vi "Oxford-1820-Main.vi"() -> ()   [LabVIEW 2013, in "Mercury iXX.lvlib"]
uses:
  <instrlib>/Mercury iXX/Mercury iXX.lvlib
  <instrlib>/Mercury iXX/Public/Controls/Unit String.ctl
  <instrlib>/Mercury iXX/Public/Libraries/Temperature/Controls/Temperature Device (Read).ctl
  <instrlib>/Mercury iXX/Public/Controls/Manufacturing Data.ctl
  <instrlib>/Mercury iXX/Public/Libraries/Temperature/Controls/Temperature Sensor Type.ctl
  <instrlib>/Mercury iXX/Public/Libraries/Temperature/Controls/Excitation Cluster.ctl
  <instrlib>/Mercury iXX/Public/Libraries/Temperature/Controls/Excitation Type.ctl
  <instrlib>/Mercury iXX/Public/Libraries/Temperature/Controls/Calibration Cluster.ctl
  <instrlib>/Mercury iXX/Public/Libraries/Temperature/Controls/Calibration Interpolation.ctl
  <instrlib>/Mercury iXX/Public/Libraries/Temperature/Controls/Loop Cluster.ctl
  <instrlib>/Mercury iXX/Public/Libraries/Temperature/Controls/Temperature Signals Cluster.ctl
  <instrlib>/Mercury iXX/Public/Libraries/Heater/Controls/Heater Device (Read).ctl
  <instrlib>/Mercury iXX/Public/Libraries/Heater/Controls/Heater Signals Cluster.ctl
  <instrlib>/Mercury iXX/Public/Libraries/Level Meter/Controls/Level Meter (Read).ctl
  <instrlib>/Mercury iXX/Public/Libraries/Level Meter/Controls/Nitrogen Configuration.ctl
  <instrlib>/Mercury iXX/Public/Libraries/Level Meter/Controls/Frequency Configuration.ctl
  <instrlib>/Mercury iXX/Public/Libraries/Level Meter/Controls/Signals.ctl
  <instrlib>/Mercury iXX/Public/Libraries/Level Meter/Controls/Helium Configuration.ctl
  <instrlib>/Mercury iXX/Public/Libraries/Level Meter/Controls/Resistance Configuration.ctl
  <instrlib>/Mercury iXX/Public/Libraries/Level Meter/Controls/Pre-Pulse.ctl
  <instrlib>/Mercury iXX/Public/Libraries/Level Meter/Controls/Pulse.ctl
  <instrlib>/Mercury iXX/Public/Libraries/Auxiliary/Controls/AUX Device (Read).ctl
  <instrlib>/Mercury iXX/Public/Libraries/Auxiliary/Controls/AUX Signals (Read).ctl
  <instrlib>/Mercury iXX/Public/Libraries/Magnet/Controls/Device (Read).ctl
  <instrlib>/Mercury iXX/Public/Libraries/Magnet/Controls/Signals (Read).ctl
  <instrlib>/Mercury iXX/Public/Libraries/Magnet/Controls/Identifier.ctl
  <instrlib>/Mercury iXX/Public/Libraries/Pressure/Controls/Pressure Device (Read).ctl
  <instrlib>/Mercury iXX/Public/Libraries/Pressure/Controls/Pressure Sensor Type.ctl
  <instrlib>/Mercury iXX/Public/Libraries/Pressure/Controls/Calibration Cluster.ctl
  <instrlib>/Mercury iXX/Public/Libraries/Pressure/Controls/Calibration Interpolation.ctl
  <instrlib>/Mercury iXX/Public/Libraries/Pressure/Controls/Loop Cluster.ctl
  <instrlib>/Mercury iXX/Public/Libraries/Pressure/Controls/Pressure Signals Cluster.ctl
  <instrlib>/Mercury iXX/Public/Libraries/Magnet/Controls/PSU Actions.ctl
  <instrlib>/Mercury iXX/Public/Libraries/Magnet/Controls/Switch Heater.ctl
  <instrlib>/Mercury iXX/Private/Controls/Command Verbs.ctl
  <instrlib>/Mercury iXX/Public/Controls/ISOBus Address.ctl
  <instrlib>/Mercury iXX/Public/Controls/Comms Transport Layer.ctl
  <instrlib>/Mercury iXX/Private/Controls/Query Dynamic Reference.ctl
  <instrlib>/Mercury iXX/Public/Controls/Mercury Reference.ctl
  <instrlib>/Mercury iXX/Public/Libraries/Magnet/Open/Open Magnet Device.vi
  <instrlib>/Mercury iXX/Public/Libraries/Magnet/Configuration/Set/PSU Action Status (Set).vi
  <instrlib>/Mercury iXX/Public/Libraries/Magnet/Signals/Read/Current (Read).vi
  <instrlib>/Mercury iXX/Public/Libraries/Magnet/Signals/Read/Persistant Current (Read).vi
  <instrlib>/Mercury iXX/Public/Libraries/Magnet/Signals/Read/Switch Heater Status (Read).vi
  <instrlib>/Mercury iXX/Public/Libraries/Magnet/Signals/Set/Switch Heater No Check (Set).vi
  <instrlib>/Mercury iXX/Public/Libraries/System/Read/Time (Read).vi
  <instrlib>/Mercury iXX/Public/Libraries/Magnet/Signals/Set/Target Field Rate (Set).vi
  <instrlib>/Mercury iXX/Public/Libraries/Magnet/Signals/Set/Target Field (Set).vi
  <instrlib>/Mercury iXX/Public/Libraries/Level Meter/Open/Open Level Meter Device.vi
  <instrlib>/Mercury iXX/Public/Libraries/Temperature/Open/Open Temperature Device.vi
  <userlib>/_OpenG.lib/error/error.llb/Filter Error Codes (Array)__ogtk.vi
  <instrlib>/Mercury iXX/Public/Libraries/System/Open/Open System.vi
  <instrlib>/Mercury iXX/Public/Libraries/System/Read/Catalogue (Read).vi
  <instrlib>/Mercury iXX/Public/Libraries/System/Read/Display Automatic Dimming (Read).vi
  <instrlib>/Mercury iXX/Public/Libraries/System/Read/Display Automatic Dimming Time (Read).vi
  <instrlib>/Mercury iXX/Public/Libraries/System/Read/Display Brightness (Read).vi
  <instrlib>/Mercury iXX/Public/Libraries/System/Read/Date (Read).vi
  <instrlib>/Mercury iXX/Public/Libraries/System/Read/DateTime (Read).vi
  <instrlib>/Mercury iXX/Public/Libraries/System/Read/HVer (Read).vi
  <instrlib>/Mercury iXX/Public/Libraries/System/Read/FVer (Read).vi
  <instrlib>/Mercury iXX/Public/Libraries/System/Read/Serial Number (Read).vi
  <instrlib>/Mercury iXX/Public/Libraries/System/Read/Flash Space (Read).vi
  <instrlib>/Mercury iXX/Public/Libraries/System/Read/Mode (Read).vi
  <instrlib>/Mercury iXX/Public/Libraries/System/Set/DateTime (Set).vi
  <instrlib>/Mercury iXX/Public/Libraries/Temperature/Configuration/Read/Serial Number (Read).vi
  <instrlib>/Mercury iXX/Public/Libraries/Temperature/Configuration/Read/Nickname (Read).vi
  <instrlib>/Mercury iXX/Public/Libraries/Temperature/Configuration/Read/Excitation Magnitude (Read).vi
  <instrlib>/Mercury iXX/Public/Libraries/Temperature/Configuration/Read/Temperature Sensor (Read).vi
  <instrlib>/Mercury iXX/Public/Libraries/Temperature/Configuration/Read/Excitation Type (Read).vi
  <instrlib>/Mercury iXX/Public/Libraries/Temperature/Configuration/Read/Calibration Hot Limit (Read).vi
  <instrlib>/Mercury iXX/Public/Libraries/Temperature/Configuration/Read/Calibration Cold Limit (Read).vi
  <instrlib>/Mercury iXX/Public/Libraries/Temperature/Signals/Read/Voltage (Read).vi
  <instrlib>/Mercury iXX/Public/Libraries/Temperature/Signals/Read/Temperature (Read).vi
  <instrlib>/Mercury iXX/Public/Libraries/Temperature/Configuration/Read/Temperature Device (Read).vi
  <instrlib>/Mercury iXX/Public/Libraries/Control Loop/Configuration/Read/Control Loop (Read).vi
  <instrlib>/Mercury iXX/Public/Libraries/Heater/Open/Open Heater Device.vi
  <instrlib>/Mercury iXX/Public/Libraries/Heater/Configuration/Read/Heater Device (Read).vi
  <instrlib>/Mercury iXX/Public/Libraries/Heater/Configuration/Read/Nickname (Read).vi
  <instrlib>/Mercury iXX/Public/Libraries/Heater/Configuration/Read/Serial Number (Read).vi
  <instrlib>/Mercury iXX/Public/Libraries/Heater/Configuration/Read/Voltage Limit (Read).vi
  <instrlib>/Mercury iXX/Public/Libraries/Heater/Configuration/Read/Nominal Resistance (Read).vi
  <instrlib>/Mercury iXX/Public/Libraries/Heater/Configuration/Read/Maximum Power (Read).vi
  <instrlib>/Mercury iXX/Public/Libraries/Heater/Signals/Read/Voltage (Read).vi
  <instrlib>/Mercury iXX/Public/Libraries/Heater/Signals/Read/Power (Read).vi
  <instrlib>/Mercury iXX/Public/Libraries/Heater/Signals/Read/Current (Read).vi
  <instrlib>/Mercury iXX/Public/Libraries/Auxiliary/Open/Open Auxiliary Device.vi
  <instrlib>/Mercury iXX/Public/Libraries/Auxiliary/Configuration/Read/Aux Device (Read).vi
  <instrlib>/Mercury iXX/Public/Libraries/Auxiliary/Configuration/Read/Serial Number (Read).vi
  <instrlib>/Mercury iXX/Public/Libraries/Auxiliary/Configuration/Read/Minimum Gas Flow (Read).vi
  <instrlib>/Mercury iXX/Public/Libraries/Auxiliary/Configuration/Read/Gas Flow Scaling (Read).vi
  <instrlib>/Mercury iXX/Public/Libraries/Auxiliary/Configuration/Read/Temperature Error Sensitivity (Read).vi
  <instrlib>/Mercury iXX/Public/Libraries/Auxiliary/Configuration/Read/Temperature Error Voltage Sensitivity (Read).vi
  <instrlib>/Mercury iXX/Public/Libraries/Auxiliary/Configuration/Read/Valve Gearing (Read).vi
  <instrlib>/Mercury iXX/Public/Libraries/Auxiliary/Configuration/Read/Stepper Speed (Read).vi
  <instrlib>/Mercury iXX/Public/Libraries/Auxiliary/Signals/Read/Position (Read).vi
  <instrlib>/Mercury iXX/Public/Libraries/Auxiliary/Signals/Read/Percent Open (Read).vi
  <instrlib>/Mercury iXX/Public/Libraries/Pressure/Open/Open Pressure Device.vi
  <instrlib>/Mercury iXX/Public/Libraries/Pressure/Configuration/Read/Pressure Device (Read).vi
  <instrlib>/Mercury iXX/Public/Libraries/Pressure/Configuration/Read/Nickname (Read).vi
  <instrlib>/Mercury iXX/Public/Libraries/Pressure/Signals/Read/Current (Read).vi
  <instrlib>/Mercury iXX/Public/Libraries/Pressure/Signals/Read/Voltage (Read).vi
  <instrlib>/Mercury iXX/Public/Libraries/Level Meter/Configuration/Read/Level Meter Device (Read).vi
  <instrlib>/Mercury iXX/Public/Libraries/Level Meter/Configuration/Read/Serial Number (Read).vi
  <instrlib>/Mercury iXX/Public/Libraries/Level Meter/Configuration/Read/Helium Probe Resistance (Read).vi
  <instrlib>/Mercury iXX/Public/Libraries/Level Meter/Configuration/Read/Helium Pulse Mag (Read).vi
  <instrlib>/Mercury iXX/Public/Libraries/Level Meter/Configuration/Read/Helium Pulse Duration (Read).vi
  <instrlib>/Mercury iXX/Public/Libraries/Level Meter/Configuration/Read/Nitrogen Freq at 100 (Read).vi
  <instrlib>/Mercury iXX/Public/Libraries/Level Meter/Configuration/Read/Nitrogen Pulse Count Period (Read).vi
  <instrlib>/Mercury iXX/Public/Libraries/Level Meter/Signals/Read/Probe Resistance Helium (Read).vi
  <instrlib>/Mercury iXX/Public/Libraries/Level Meter/Signals/Read/Probe Level Helium (Read).vi
  <instrlib>/Mercury iXX/Public/Libraries/Level Meter/Signals/Read/Probe Count Nitrogen (Read).vi
  <instrlib>/Mercury iXX/Public/Libraries/Level Meter/Signals/Read/Probe Level Nitrogen (Read).vi
  <instrlib>/Mercury iXX/Public/Libraries/Magnet/Configuration/Read/Magnet Device (Read).vi
  <instrlib>/Mercury iXX/Public/Libraries/Magnet/Configuration/Read/Serial Number (Read).vi
  <instrlib>/Mercury iXX/Public/Libraries/Magnet/Configuration/Read/Bipolar Output (Read).vi
  <instrlib>/Mercury iXX/Public/Libraries/Magnet/Configuration/Read/Output Configuration (Read).vi
  <instrlib>/Mercury iXX/Public/Libraries/Magnet/Configuration/Read/Current Limit (Read).vi
  <instrlib>/Mercury iXX/Public/Libraries/Magnet/Configuration/Read/Current to Field Factor (Read).vi
  <instrlib>/Mercury iXX/Public/Libraries/Magnet/Configuration/Read/Switch Present (Read).vi
  <instrlib>/Mercury iXX/Public/Libraries/Magnet/Configuration/Read/Software Voltage Limit (Read).vi
  <instrlib>/Mercury iXX/Public/Libraries/Magnet/Signals/Read/Current Rate (Read).vi
  <instrlib>/Mercury iXX/Public/Libraries/Magnet/Configuration/Read/PSU Action Status (Read).vi
  <instrlib>/Mercury iXX/Public/Libraries/Magnet/Signals/Read/Voltage (Read).vi
  <instrlib>/Mercury iXX/Public/Libraries/Magnet/Signals/Read/Field (Read).vi
  <instrlib>/Mercury iXX/Public/Libraries/Magnet/Signals/Read/Target Field Rate (Read).vi
  <instrlib>/Mercury iXX/Public/Libraries/Magnet/Signals/Read/Target Field (Read).vi
  <instrlib>/Mercury iXX/Public/Libraries/Magnet/Signals/Read/Persistant Field (Read).vi
  <instrlib>/Mercury iXX/Public/Libraries/Pressure.lvlib
  <instrlib>/Mercury iXX/Public/Libraries/System.lvlib
  <instrlib>/Mercury iXX/Public/Libraries/Control Loop.lvlib
  <instrlib>/Mercury iXX/Public/Libraries/Heater.lvlib
  <instrlib>/Mercury iXX/Public/Libraries/Temperature.lvlib
  <instrlib>/Mercury iXX/Public/Libraries/Auxiliary.lvlib
  <instrlib>/Mercury iXX/Public/Libraries/Magnet.lvlib
  <instrlib>/Mercury iXX/Public/Libraries/Level Meter.lvlib
  <instrlib>/Mercury iXX/Public/Libraries/System/Open/Open Device.vi
panel:
  out "LPF ON":timestamp
  in  "Tab Control":T1(tab)
  out "LPF Pressure":dbl format="%_5f mB"
  out "LPF Needle Valve (%)":dbl format="%_6g"
  out "LPF Temperature":dbl=4.2075 format="%_2f K"
  out "Magnet Temperature":dbl=3.8705 format="%_2f K"
  in  "Set Needle Valve (%)":dbl format="%_2g"
  out "He LVL Chart":dbl(slide)=52.0833 scale=0.0..100.0
  out "N2 LVL Chart":dbl(slide)=61.3025 scale=0.0..100.0
  out "Sentinel":bool=TRUE
  in  "Remote Mode":bool
  out "Power Supply Field (T)":dbl=0.0001 format="%#.5f"
  out "Magnet Field (T)":dbl format="%.5f"
  out "Voltage (V)":dbl=-0.0003 format="%.5f"
  out "Current (A)":dbl=0.0006 format="%.5f"
  out "N2 LEVEL":dbl=61.3025 format="%.0f %"
  out "He LEVEL":dbl=52.0833 format="%.0f %"
  in  "Fast/Slow Fill":bool
  in  "OK":bool
  out "Magnet Field (T)":dbl(knob) caption="Voltage (V)" scale=-20.0..20.0
  out "Magnet Status 2":string
  out "Switch Time":string="11:11:48"
  out "SWITCH HEATER":bool
  in  "PS Heat":bool
  in  "Clamp":bool
  in  "To Set":bool
  in  "To Zero":bool
  in  "Hold":bool
  out "Magnet Status":string="Clamped"
  out "Target Field Rate (T/min)":dbl=1.0 format="%.5f"
  out "Target Field (T)":dbl format="%#.5f"
  in  "Target Rate (T/min)":dbl=0.1 format="%.5f"
  in  "Target Field (T)":dbl format="%#.5f"
  in  "Send to IPS":bool
  out "Voltage (V)":dbl(knob)=-0.0003 scale=-10.0..10.0
  out "Current (A)":dbl(knob)=0.0006 scale=-180.0..180.0
  in  "Mercury Functions":T2(tab)=enum."Temperature"
  out "time stamp":timestamp=timestamp(3543841780 s since 1904-01-01)
  out "Free Space":i32=166384 caption="Free Space (KB)"
  out "Set Date Response":string="VALID"
  out "String":string="NORM" caption="User Mode"
  out "Date":string="2016:04:18"
  out "Time":string="11:29:40"
  out "Hardware Version":string="65"
  out "Firmware Version":string="2.2.6.20"
  out "Serial Number":string="154650110"
  out "ITC Devices":string[](array[string])=["DB4.G1:AUX", "DB8.P1:PRES", "MB0.H1:HTR", "MB1.T1:TEMP"]
  out "S/W Version(s)":string[](array[string])=["2.2.6.20\n"]
  out "Serial Number(s)":string[](array[string])=["154650110"]
  out "# of Instruments":i32=1
  out "Automatic Dimming":string="OFF"
  out "Dimming Time":string="5"
  out "Display Brightness":string="100"
  in  "ITC IP Address":string="130.49.180.101"
  out "Excitation Magnitude":dbl=5.0
  out "Sensor Type":string="NTC"
  out "Excitation Type":string="UNIP"
  out "Hot Limit":dbl=1000.0
  out "H Unit":T3="K"
  out "Cold Limit":dbl=1000.0
  out "C Unit":T3="K"
  out "Unit":T3
  out "Voltage":dbl=0.005
  out "V Unit":T3="V"
  out "Temperature":dbl=4.2075
  out "T Unit":T3="K"
  out "Temperature Device Settings":T4={"Manufacturing"={"Hardware Version"="65", "Firmware Version"="2.2", "Serial Number"="154650110"}, "Temperature Sensor Type"="NTC", "Excitation"={"Excitation Type"="UNIP", "Magnitude"="5.00"}, "Calibration"={"Filename"="59543_iTC-lambda.dat", "Interpolation"="LIN", "Scaling Factor"="1", "Offset Factor"="0", "Hot Limit"="1000.00K", "Cold Limit"="1000.00K", "Last Calibration"="", "Reference"="Internal"}, "Control Loop"={"Heater"="", "Auxiliary"="", "Heater Auto"="", "Percentage Heat"="", "Temperature Set Point"="", "PID Auto (from file)"="", "P Value"="", "I Value"="", "D Value"="", "Auto PID Table Filename"="", "Flow Auto"="", "Target Heater Table"="", "Sweep mode"="", "Sweep Table Filename"="", "Percentage Flow"=""}, "Temperature Signals"={"Voltage"="5.0000mV", "Current"="3.9694µA", "Power"="0.0199µW", "Resistance"="1259.6510R", "Temperature"="4.2075K", "Sensitivity"="299.3801R/K", "Reference"="N/A"}, "Nickname"="Mag_AB_MB1", "Status"="0"}
  out "Temp S/N":string="154650110"
  out "T Nickname":string="Mag_AB_MB1"
  out "T Loop Details":T11
  out "Heater Device Settings":T13={"Manufacturing"={"Hardware Version"="65", "Firmware Version"="2.3", "Serial Number"="154650110"}, "Nickname"="MB0.H1", "Voltage Limit"="1", "Nominal Resistance"="10", "Maximum Power"="0.1000", "Heater Signals"={"Voltage"="0.0507V", "Current"="-0.0000A", "Power"="0.0000W"}, "Status"="2"}
  out "Htr C Unit":T3="A"
  out "Htr P Unit":T3="W"
  out "Htr V Unit":T3="V"
  out "Htr Current":dbl=-0.0
  out "Htr Power":dbl
  out "Htr Voltage":dbl=0.0507
  out "Power Unit":T3
  out "Volt Unit":T3
  out "Res Unit":T3
  out "Maximum Power":dbl=0.1
  out "Htr Resistance":dbl=10.0
  out "Htr Voltage Limit":dbl=1.0
  out "Htr S/N":string="154650110"
  out "Htr Nickname":string="MB0.H1"
  out "Pressure Device":T15={"Manufacturing"={"Hardware Version"="3", "Firmware Version"="1.10", "Serial Number"="151150091"}, "Temperature Sensor Type"="RAT", "Calibration"={"Filename"="Lambda pressure control_10V ratiometric.dat", "Interpolation"="LIN", "Scaling Factor"="1", "Offset Factor"="-0.0004", "High Limit"="1000.00K", "Low Limit"="1000.00K", "Last Calibration"=""}, "Control Loop"={"Heater"="None", "Auxiliary"="None", "Heater Auto"="", "Percentage Heat"="", "Pressure Set Point"="", "PID Auto (from file)"="", "P Value"="", "I Value"="", "D Value"="1.0", "Auto PID Table Filename"="", "Flow Auto"="", "Target Heater Table"="", "Sweep mode"="", "Sweep Table Filename"="", "Percentage Flow"=""}, "Pressure Signals"={"Voltage"="-0.0822mV", "Current"="-0.0000A", "Power"="0.0000W", "Pressure"="0.0000mB"}, "Nickname"="Lam_P_DB8", "Status"="0"}
  out "Nickname":string="Lam_P_DB8"
  out "Current":dbl=-0.0
  out "Voltage":dbl=-8.219999999999999e-05
  out "Auxiliary Device Details":T21={"Manufacturing"={"Hardware Version"="65", "Firmware Version"="3.1", "Serial Number"="154650084"}, "Min Flow"=0.0, "Scaling Factor"=50.0, "Temp Err"=9.0, "Temp V Err"=11.0, "Gear"=2, "Speed"=2, "Signals"={"Position"=0.0, "% Open"=0.0, "I0"="ON", "I1"="OFF", "I2"="OFF", "I3"="OFF", "O0"="OFF", "O1"="OFF", "O2"="OFF", "O3"="OFF"}, "Nickname"="DB4.G1", "Status"="0"} {"Signals"."% Open" min=0.0 max=100.0 step=0.1 format="%.4f"; "Signals"."Position" max=20.0 step=1.0 format="%.4f"; "Speed" max=7 step=1; "Gear" max=7 step=1; "Temp V Err" min=0.0 max=20.0 step=0.1; "Temp Err" min=0.0 max=20.0 step=0.1; "Scaling Factor" min=0.0 max=99.0 step=0.1; "Min Flow" min=0.0 max=20.0 step=0.1}
  out "Aux S/N":string="154650084"
  out "Min Flow":dbl caption="Minimum Gas Flow" format="%#.1f"
  out "Scaling Factor":dbl=50.0 caption="Gas Flow Scaling Factor" format="%#.1f"
  out "Temp Err":dbl=9.0 caption="Temperature Error Sensitivity" format="%#.1f"
  out "Temp V Err":dbl=11.0 caption="Temperature Voltage Error Sensitivity" format="%#.1f"
  out "Gear":u32=2 caption="Valve Gearing"
  out "Speed":u32=2 caption="Stepper Speed"
  out "Unit 2":T3
  out "Unit 3":T3
  out "Unit 4":T3
  out "Unit 5":T3
  out "Unit 6":T3
  out "Unit 7":T3
  out "Position":u32
  out "% Open":dbl caption="Percentage Open (%)"
  out "Unit":T3
  out "Unit":T3="%"
  out "time stamp 2":timestamp=timestamp(3543841781 s since 1904-01-01)
  out "Free Space 2":i32=166316 caption="Free Space (KB)"
  out "Set Date Response 2":string="VALID"
  out "String 2":string="NORM" caption="User Mode"
  out "Date 2":string="2016:04:18"
  out "Time 2":string="11:29:45"
  out "Hardware Version 2":string="65"
  out "Firmware Version 2":string="2.2.6.20"
  out "Serial Number 2":string="153350063"
  out "IPS Devices":string[](array[string])=["DB3.L1:LVL", "GRPX:PSU", "GRPY:PSU", "GRPZ:PSU", "MB1.T1:TEMP", "PSU.M1:PSU", "PSU.M2:PSU", "PSU.M3:PSU"]
  out "S/W Version(s) 2":string[](array[string])=["2.2.6.20\n"]
  out "Serial Number(s) 2":string[](array[string])=["153350063"]
  out "# of Instruments 2":i32=1
  out "Automatic Dimming 2":string="OFF"
  out "Dimming Time 2":string="5"
  out "Display Brightness 2":string="100"
  in  "IPS IP Address":string="130.49.180.102"
  out "LVL Device DetailSettings":T23={"Manufacturing"={"Hardware Version"="65", "Firmware Version"="2.2", "Serial Number"="152450013"}, "Nitrogen Configuration"={"Frequency Configuration"={"Freq 0%"=0.0, "Freq 100%"=0.0}, "Pulse Period"=0.0}, "Signals"={"Helium Signals"={"Resistance"=75.5626, "Level"=52.0833}, "Nitrogen Signals"={"Count"=8800.0, "Freq"=487361.0, "Level"=61.3445}}, "Nickname"="DB3.L1", "Status"="0", "Helium Configuration"={"Resistance Configuration"={"Res 0%"=0.0, "Res 100%"=0.0}, "Pre-Pulse"={"Magnitude"=0.0, "Duration"=0.0}, "Pulse"={"Magnitude"=0.0, "Duration"=0.0, "Delay"=0.0}}}
  out "LVL S/N":string="152450013"
  out "LVL P Magnitude":dbl=125.0 caption="Pulse Magnitude (mA)"
  out "LVL P Duration":dbl=5.0 caption="Pulse Duration (s)"
  out "N Freq 100%":dbl=7880.0 caption="Frequency at 100% (Hz)"
  out "N Pulse Period":dbl=1000.0 caption="Pulse Period (ms)"
  out "He Res Config":T28={"Res 0%"=149.0, "Res 100%"=8.0}
  out "He Resistance":dbl=75.5626 caption="Resistance (Ohms)"
  out "He Level":dbl=52.0833 caption="Helium Level (%)"
  out "N Counter":u32 caption="Counter"
  out "N Level":dbl=61.3445 caption="Nitrogen Level (%)"
  out "Excitation Magnitude 2":dbl=5.0
  out "Sensor Type 2":string="NTC"
  out "Excitation Type 2":string="UNIP"
  out "Hot Limit 2":dbl=1000.0
  out "H Unit 2":T3="K"
  out "Cold Limit 2":dbl=1000.0
  out "C Unit 2":T3="K"
  out "Unit 12":T3
  out "Voltage 2":dbl=0.005
  out "V Unit 2":T3="V"
  out "Temperature 2":dbl=3.8706
  out "T Unit 2":T3="K"
  out "Temperature Device Settings 2":T4={"Manufacturing"={"Hardware Version"="65", "Firmware Version"="2.2", "Serial Number"="153350063"}, "Temperature Sensor Type"="NTC", "Excitation"={"Excitation Type"="UNIP", "Magnitude"="5.00"}, "Calibration"={"Filename"="Bob.dat", "Interpolation"="LIN", "Scaling Factor"="1", "Offset Factor"="0", "Hot Limit"="1000.00K", "Cold Limit"="1000.00K", "Last Calibration"="", "Reference"="Internal"}, "Control Loop"={"Heater"="", "Auxiliary"="", "Heater Auto"="", "Percentage Heat"="", "Temperature Set Point"="", "PID Auto (from file)"="", "P Value"="", "I Value"="", "D Value"="", "Auto PID Table Filename"="", "Flow Auto"="", "Target Heater Table"="", "Sweep mode"="", "Sweep Table Filename"="", "Percentage Flow"=""}, "Temperature Signals"={"Voltage"="5.0000mV", "Current"="3.5897µA", "Power"="0.0179µW", "Resistance"="1392.8897R", "Temperature"="3.8706K", "Sensitivity"="359.8580R/K", "Reference"="N/A"}, "Nickname"="MB1.T1", "Status"="0"}
  out "Temp S/N 2":string="153350063"
  out "T Nickname 2":string="MB1.T1"
  out "T Loop Details 2":T11
  out "Magnet Device Details":T31={"Manufacturing"={"Hardware Version"="NOT_FOUND", "Firmware Version"="NOT_FOUND", "Serial Number"="NOT_FOUND"}, "Nickname"="GRPZ", "Bipolar Output"="ON", "String"="PARA", "Current Limit"=174.0, "AtoB"=8.688, "Inductance"=39.406, "Switch Present"="PSU.M1", "Swh Htr Current"=86.0, "SW VLIM"=9.0, "V Trans Time"=1000.0, "Magnet PSU Signals"={"Voltage"=-0.0002, "Current"=0.0002, "Current Rate"=100.0, "Field"=0.0001, "Field Rate"=11.5101, "Persistant Current"=0.0003, "Persistant Field"=0.0, "Target Current"=0.0, "Target Field"=0.0, "Target Current Rate"=8.688, "Target Field Rate"=1.0, "Switch Heater Status (SWHT)"="OFF", "Switch Heater Status (SWHN)"="OFF"}, "PSU Action"="CLMP", "Status"="40000000", "Level Limit"=0.0, "Temperature Limit"=999.0} {"Temperature Limit" format="%#.1f"; "Level Limit" format="%#.1f"; "V Trans Time" format="%#.1f"; "SW VLIM" format="%#.1f"; "Swh Htr Current" format="%#.1f"; "Inductance" format="%#.1f"; "AtoB" format="%#.1f"; "Current Limit" format="%#.1f"}
  out "Mag S/N":string="NOT_FOUND"
  out "Bipolar Output":string="ON"
  out "Out Config":string="PARA" caption="Output Configuration"
  out "Current Limit":dbl=174.0 caption="Current Limit (A)" format="%#.1f"
  out "AtoB":dbl=8.688 caption="Current Field Factor (A/T)" format="%#.1f"
  out "Switch Present":string="PSU.M1"
  out "SW VLIM":dbl=9.0 caption="Software Voltage Limit (V)" format="%#.1f"
  out "Unit 8":T3
  out "Unit 9":T3
  out "Unit 10":T3
  out "Current Rate":dbl=100.0
  out "PSU Act Stat":string="CLMP" caption="PSU Action Status"
  out "Unit 11":T3="A/min"
  in  "Device Identifier":T33="GRPZ"
  out "Error List":T34(array[cluster])
  in  "Lambda":bool
  out "LPF on (s)":i32=5373
  # "Voltage (V)"
  # "Magnet (T)"
  # "Current (A)"
  # "Slow Rates\nCurrent Range (A)     Field Range (T)    Rate (T/min)\n0       -- 100        0    -- 11.5       0.91\n100     -- 150        11.5 -- 17.2       0.23\n150     -- 155.467    17.2 -- 18         0.11\n155.567 -- 172.471    18   -- 20         0.11\n\nFast Rates\nCurrent Range (A)     Field Range (T)    Rate (T/min)\n0       -- 155.467    0    -- 18         1.0\n155.567 -- 172.471    18   -- 20         0.25"
  # "ITC: 101\nIPS: 102\nIPS VR: 67"
  # "ITC: 101\nIPS: 102\nIPS VR: 67"
  # "This Control Doesn't Work"
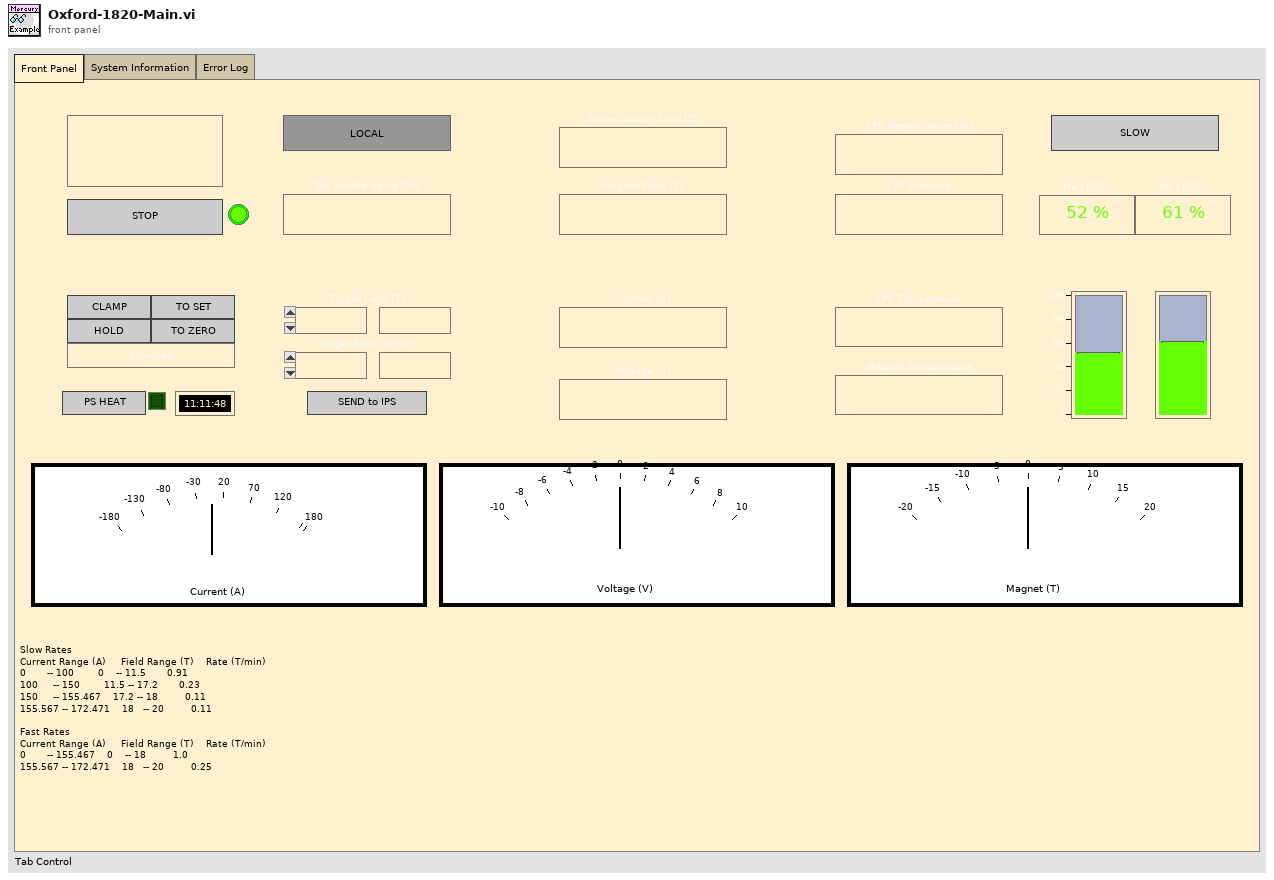
[diagram p1: front panel]
types:
  T1 = enum32{"Front Panel", "System Information", "Error Log"}
  T2 = enum32{"System: ITC", "Temperature", "Heater", "Pressure", "Auxiliary", "System: IPS", "Level Meter", "Temperature 2", "Magnet"}
  T3 = typedef "Mercury iXX.lvlib/Unit String.ctl" = string
  T4 = typedef "Mercury iXX.lvlib/Temperature.lvlib/Temperature Device (Read).ctl" = cluster{"Manufacturing":T5, "Temperature Sensor Type":T6, "Excitation":T7, "Calibration":T9, "Control Loop":T11, "Temperature Signals":T12, "Nickname":string, "Status":string}
  T5 = typedef "Mercury iXX.lvlib/Manufacturing Data.ctl" = cluster{"Hardware Version":string, "Firmware Version":string, "Serial Number":string}
  T6 = typedef "Mercury iXX.lvlib/Temperature.lvlib/Temperature Sensor Type.ctl" = string
  T7 = typedef "Mercury iXX.lvlib/Temperature.lvlib/Excitation Cluster.ctl" = cluster{"Excitation Type":T8, "Magnitude":string}
  T8 = typedef "Mercury iXX.lvlib/Temperature.lvlib/Excitation Type.ctl" = string
  T9 = typedef "Mercury iXX.lvlib/Temperature.lvlib/Calibration Cluster.ctl" = cluster{"Filename":string, "Interpolation":T10, "Scaling Factor":string, "Offset Factor":string, "Hot Limit":string, "Cold Limit":string, "Last Calibration":string, "Reference":string}
  T10 = typedef "Mercury iXX.lvlib/Temperature.lvlib/Calibration Interpolation.ctl" = string
  T11 = typedef "Mercury iXX.lvlib/Temperature.lvlib/Loop Cluster.ctl" = cluster{"Heater":string, "Auxiliary":string, "Heater Auto":string, "Percentage Heat":string, "Temperature Set Point":string, "PID Auto (from file)":string, "P Value":string, "I Value":string, "D Value":string, "Auto PID Table Filename":string, "Flow Auto":string, "Target Heater Table":string, "Sweep mode":string, "Sweep Table Filename":string, "Percentage Flow":string}
  T12 = typedef "Mercury iXX.lvlib/Temperature.lvlib/Temperature Signals Cluster.ctl" = cluster{"Voltage":string, "Current":string, "Power":string, "Resistance":string, "Temperature":string, "Sensitivity":string, "Reference":string}
  T13 = typedef "Mercury iXX.lvlib/Heater.lvlib/Heater Device (Read).ctl" = cluster{"Manufacturing":T5, "Nickname":string, "Voltage Limit":string, "Nominal Resistance":string, "Maximum Power":string, "Heater Signals":T14, "Status":string}
  T14 = typedef "Mercury iXX.lvlib/Heater.lvlib/Heater Signals Cluster.ctl" = cluster{"Voltage":string, "Current":string, "Power":string}
  T15 = typedef "Mercury iXX.lvlib/Pressure.lvlib/Pressure Device (Read).ctl" = cluster{"Manufacturing":T5, "Temperature Sensor Type":T16, "Calibration":T17, "Control Loop":T19, "Pressure Signals":T20, "Nickname":string, "Status":string}
  T16 = typedef "Mercury iXX.lvlib/Pressure.lvlib/Pressure Sensor Type.ctl" = string
  T17 = typedef "Mercury iXX.lvlib/Pressure.lvlib/Calibration Cluster.ctl" = cluster{"Filename":string, "Interpolation":T18, "Scaling Factor":string, "Offset Factor":string, "High Limit":string, "Low Limit":string, "Last Calibration":string}
  T18 = typedef "Mercury iXX.lvlib/Pressure.lvlib/Calibration Interpolation.ctl" = string
  T19 = typedef "Mercury iXX.lvlib/Pressure.lvlib/Loop Cluster.ctl" = cluster{"Heater":string, "Auxiliary":string, "Heater Auto":string, "Percentage Heat":string, "Pressure Set Point":string, "PID Auto (from file)":string, "P Value":string, "I Value":string, "D Value":string, "Auto PID Table Filename":string, "Flow Auto":string, "Target Heater Table":string, "Sweep mode":string, "Sweep Table Filename":string, "Percentage Flow":string}
  T20 = typedef "Mercury iXX.lvlib/Pressure.lvlib/Pressure Signals Cluster.ctl" = cluster{"Voltage":string, "Current":string, "Power":string, "Pressure":string}
  T21 = typedef "Mercury iXX.lvlib/Auxiliary.lvlib/AUX Device (Read).ctl" = cluster{"Manufacturing":T5, "Min Flow":dbl, "Scaling Factor":dbl, "Temp Err":dbl, "Temp V Err":dbl, "Gear":u32, "Speed":u32, "Signals":T22, "Nickname":string, "Status":string}
  T22 = typedef "Mercury iXX.lvlib/Auxiliary.lvlib/AUX Signals (Read).ctl" = cluster{"Position":dbl, "% Open":dbl, "I0":string, "I1":string, "I2":string, "I3":string, "O0":string, "O1":string, "O2":string, "O3":string}
  T23 = typedef "Mercury iXX.lvlib/Level Meter.lvlib/Level Meter (Read).ctl" = cluster{"Manufacturing":T5, "Nitrogen Configuration":T24, "Signals":T26, "Nickname":string, "Status":string, "Helium Configuration":T27}
  T24 = typedef "Mercury iXX.lvlib/Level Meter.lvlib/Nitrogen Configuration.ctl" = cluster{"Frequency Configuration":T25, "Pulse Period":dbl}
  T25 = typedef "Mercury iXX.lvlib/Level Meter.lvlib/Frequency Configuration.ctl" = cluster{"Freq 0%":dbl, "Freq 100%":dbl}
  T26 = typedef "Mercury iXX.lvlib/Level Meter.lvlib/Signals.ctl" = cluster{"Helium Signals":cluster{"Resistance":dbl, "Level":dbl}, "Nitrogen Signals":cluster{"Count":dbl, "Freq":dbl, "Level":dbl}}
  T27 = typedef "Mercury iXX.lvlib/Level Meter.lvlib/Helium Configuration.ctl" = cluster{"Resistance Configuration":T28, "Pre-Pulse":T29, "Pulse":T30}
  T28 = typedef "Mercury iXX.lvlib/Level Meter.lvlib/Resistance Configuration.ctl" = cluster{"Res 0%":dbl, "Res 100%":dbl}
  T29 = typedef "Mercury iXX.lvlib/Level Meter.lvlib/Pre-Pulse.ctl" = cluster{"Magnitude":dbl, "Duration":dbl}
  T30 = typedef "Mercury iXX.lvlib/Level Meter.lvlib/Pulse.ctl" = cluster{"Magnitude":dbl, "Duration":dbl, "Delay":dbl}
  T31 = typedef "Mercury iXX.lvlib/Magnet.lvlib/Device (Read).ctl" = cluster{"Manufacturing":T5, "Nickname":string, "Bipolar Output":string, "String":string, "Current Limit":dbl, "AtoB":dbl, "Inductance":dbl, "Switch Present":string, "Swh Htr Current":dbl, "SW VLIM":dbl, "V Trans Time":dbl, "Magnet PSU Signals":T32, "PSU Action":string, "Status":string, "Level Limit":dbl, "Temperature Limit":dbl}
  T32 = typedef "Mercury iXX.lvlib/Magnet.lvlib/Signals (Read).ctl" = cluster{"Voltage":dbl, "Current":dbl, "Current Rate":dbl, "Field":dbl, "Field Rate":dbl, "Persistant Current":dbl, "Persistant Field":dbl, "Target Current":dbl, "Target Field":dbl, "Target Current Rate":dbl, "Target Field Rate":dbl, "Switch Heater Status (SWHT)":string, "Switch Heater Status (SWHN)":string}
  T33 = typedef "Mercury iXX.lvlib/Magnet.lvlib/Identifier.ctl" = string
  T34 = cluster{"time":timestamp, "code":i32, "source":string}[]
  T35 = cluster{"Hold":bool, "Clamp":bool, "To Set":bool, "To Zero":bool, "Send to IPS":bool, "PS Heat":bool, "Lambda":bool}
  T36 = typedef "Mercury iXX.lvlib/Magnet.lvlib/PSU Actions.ctl" = string
  T37 = typedef "Mercury iXX.lvlib/Magnet.lvlib/Switch Heater.ctl" = string
  T38 = typedef "Mercury iXX.lvlib/Command Verbs.ctl" = string
  T39 = typedef "Mercury iXX.lvlib/ISOBus Address.ctl" = i32
  T40 = enum32{"invalid app kind", "Development System", "Run Time System", "Student Edition", "Embedded LabVIEW", "Evaluation", "Custom"}
  T41 = cluster{"time":timestamp, "code":i32, "source":string}
  T42 = enum32{"Invalid", "Standard", "Closed", "Hidden", "Minimized", "Maximized"}
  T43 = cluster{"Magnet Field":dbl, "PS Field":dbl, "Target Field":dbl, "Target Field Rate":dbl, "Voltage":dbl, "Current":dbl}
  T44 = typedef "Mercury iXX.lvlib/Comms Transport Layer.ctl" = enum16{"Ethernet TCP/IP", "USB", "ISOBus - RS-232", "GPIB"}
  T45 = typedef "Mercury iXX.lvlib/Query Dynamic Reference.ctl" = refnum<vi>
  T46 = typedef "Mercury iXX.lvlib/Mercury Reference.ctl" = cluster{"Comms":refnum<visa-resource-name>, "Device ID":string[], "Comms Layer":T44, "Command":string, "Query reference":T45}
  T47 = cluster{"Core":cluster{"Current VI Reference":refnum<vi>, "Close Panel on Exit?":bool}, "Mercury ITC Ref":cluster{"Comms":refnum<visa-resource-name>, "Device ID":string[], "Comms Layer":T44, "Command":string, "Query reference":T45}, "Mercury IPS Ref":T46, "sentinel":bool, "Error Log":cluster{"time":timestamp, "code":i32, "source":string}[]}
  T48 = typedef "Mercury iXX.lvlib/Response String.ctl" = string
  T49 = cluster{"Target Field (T)":dbl, "Target Field Rate (T/min)":dbl}
  T50 = cluster{"Comms":refnum<visa-resource-name>, "Device ID":string[], "Comms Layer":T44, "Command":string, "Query reference":T45}
  T51 = typedef "Filtered Error Details - Cluster__ogtk.ctl" = cluster{"code":i32, "source":string}
  T52 = cluster{"Current VI Reference":refnum<vi>, "Close Panel on Exit?":bool}
  T53 = typedef "Mercury iXX.lvlib/System.lvlib/User Mode.ctl" = string
  T54 = typedef "Mercury iXX.lvlib/Magnet.lvlib/Output Configuration.ctl" = string
  T55 = cluster{"Magnet Field":dbl, "PS Field":dbl, "Target Field":dbl, "Target Field Rate":dbl, "Voltage":dbl, "Current":dbl, "Switch":bool}
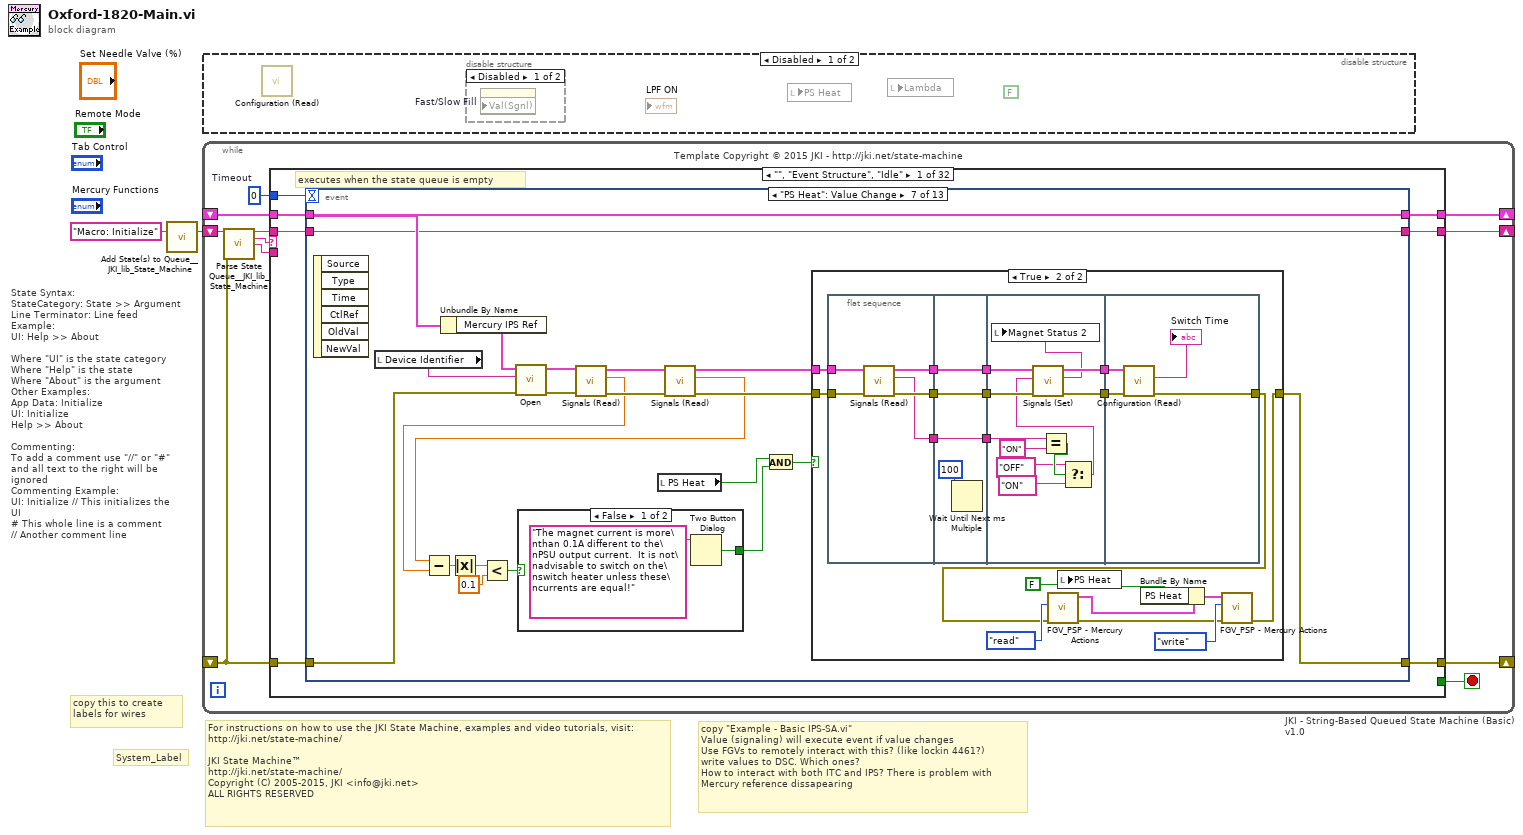
[diagram p0: block diagram]
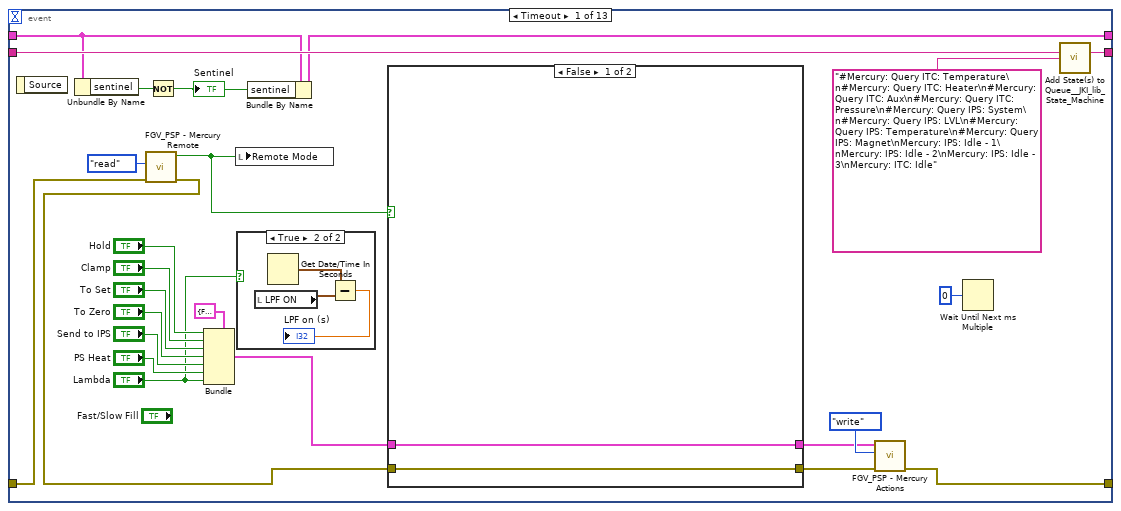
[diagram p4: hidden frame]
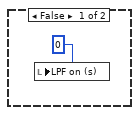
[diagram p5: hidden frame]
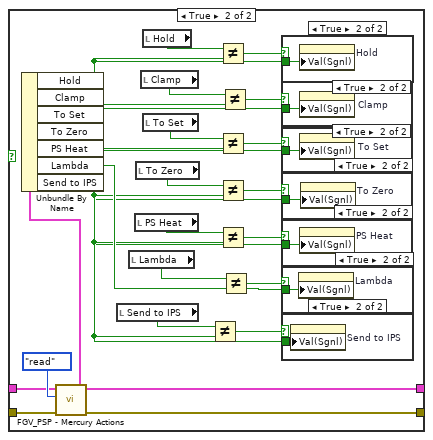
[diagram p6: hidden frame]
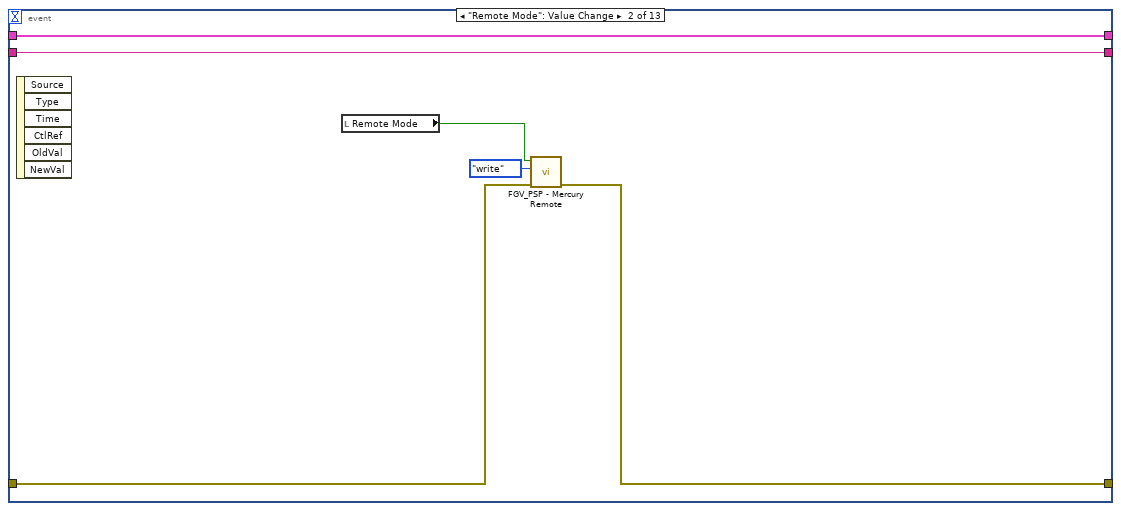
[diagram p14: hidden frame]
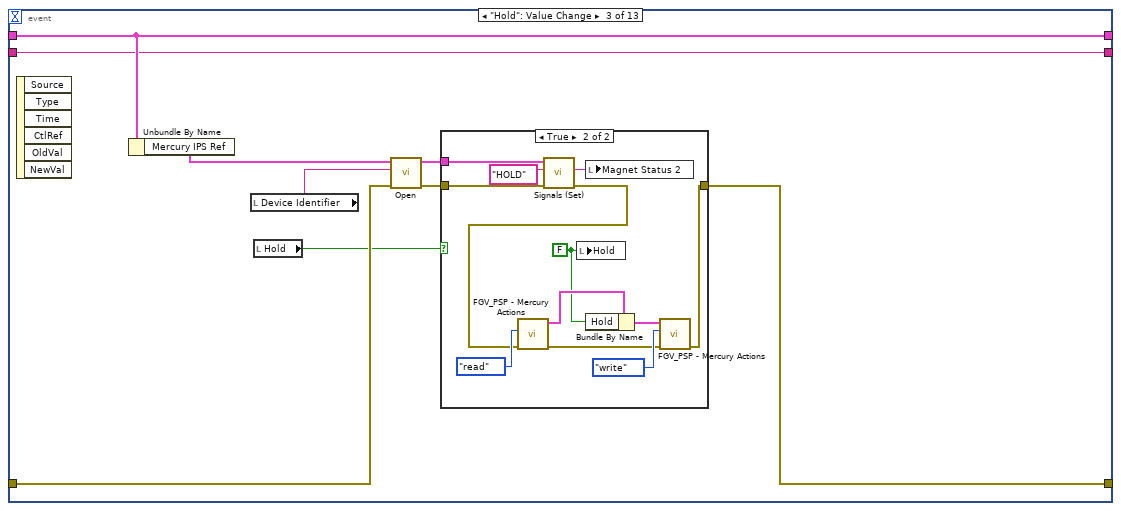
[diagram p15: hidden frame]
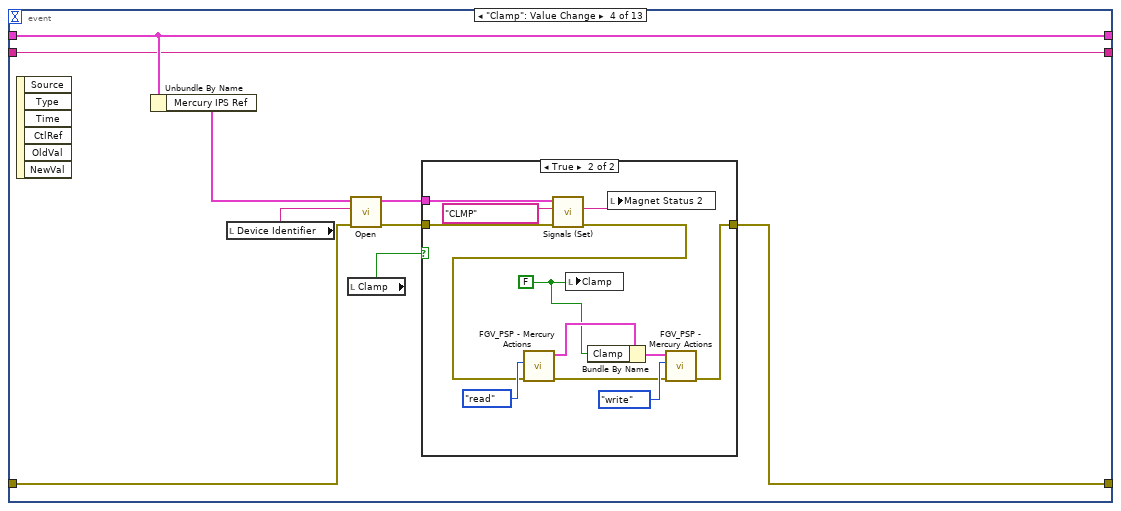
[diagram p17: hidden frame]
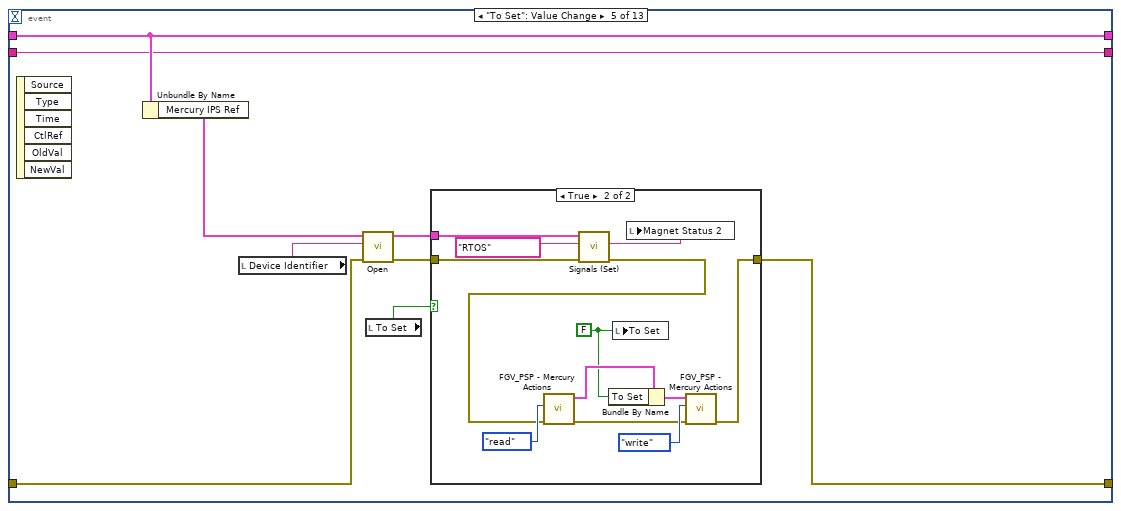
[diagram p19: hidden frame]
diagram:
  # "copy \"Example - Basic IPS-SA.vi\"\nValue (signaling) will execute event if value changes\nUse FGVs to remotely interact with this? (like lockin 4461?)\nwrite values to DSC. Which ones?\nHow to interact with both ITC and IPS? There is problem with \nMercury reference dissapearing"
  # "For instructions on how to use the JKI State Machine, examples and video tutorials, visit:\nhttp://jki.net/state-machine/\n\nJKI State Machine™\nhttp://jki.net/state-machine/\nCopyright (C) 2005-2015, JKI <info@jki.net>\nALL RIGHTS RESERVED"
  # "State Syntax:\nStateCategory: State >> Argument\nLine Terminator: Line feed\nExample:\nUI: Help >> About\n\nWhere \"UI\" is the state category\nWhere \"Help\" is the state\nWhere \"About\" is the argument\nOther Examples:\nApp Data: Initialize\nUI: Initialize\nHelp >> About\n\nCommenting:\nTo add a comment use \"//\" or \"#\" and all text to the right will be ignored\nCommenting Example:\nUI: Initialize // This initializes the UI\n# This whole line is a comment\n// Another comment line"
  # "copy this to create labels for wires"
  # "System_Label"
  n1 = call <vilib>:"Add State(s) to Queue__JKI_lib_State_Machine.vi"("State(s) in (\"\")"="Macro: Initialize") -> ("States Out"=w2:string)  [unwired: 14 in]
  n2 = while "JKI - String-Based Queued State Machine (Basic) v1.0" {
    shift-right: [w6] -> _
    shift-left: _ -> [w5]
    shift-right: [w9] -> _
    shift-left: _ -> [w3]
    shift-right: [w8] -> _
    shift-left: w2 -> [w10]
    stop <- w7 stop-if-true
    w4 = 0  # Timeout
    # "Template Copyright © 2015 JKI - http://jki.net/state-machine"
    n3 = call <vilib>:"Parse State Queue__JKI_lib_State_Machine.vi"("State Queue"=w10, "Error In (no error)"=w3) -> ("Remaining States"=w12:string, "Current State"=w13:string, "Arguments"=w11:string)  [unwired: 11 in]
    n4 = case shown="\"\", \"Event Structure\", \"Idle\"" w13 {
      selector: w13 -> [_ _ w361 _ _ _ _ _ _ _ _ _ _ _ _ _ _ _ _ _ _ _ _ _ _ _ _ _ _ _ _ _]
      tunnel: w12 -> [w20 w360 w365 w383 w400 w405 w409 w418 w424 w428 w440 w447 w458 w484 w489 w504 w508 w531 w575 w621 w663 w710 w731 w776 w817 w864 w905 w948 w1005 w1044 w1048 w1053]
      tunnel: w11 -> [_ _ _ _ _ _ _ _ _ _ _ w442 w452 _ _ _ _ _ _ _ _ _ _ _ _ _ _ _ _ _ _ _]
      tunnel: w5 -> [w16 w357 w363 w374 w386 w403 w406 _ w419 w425 w438 w445 w454 w481 w487 w502 w505 w526 w573 w620 w627 w670 w717 w774 w816 w863 w904 w947 w1004 w1043 w1047 w1052]
      tunnel: [w14 w358 w367 w380 errorcluster {"status"=FALSE, "code"=0, "source"=""} ("error out") w402 w407 w411 w420 w426 w434 w443 w455 w482 w486 w490 w506 w510 w535 w582 w624 w673 w718 w738 w783 w822 w871 w910 w982 w1017 w1046 w1050] -> w9
      tunnel: [w19 w359 w364 w382 w399 w404 w408 w417 w423 w427 w439 w446 w457 w483 w488 w503 w507 w530 w574 w622 w664 w711 w732 w775 w818 w865 w906 w949 w1006 w1045 w1049 w1054] -> w8
      tunnel: [_ _ _ _ _ TRUE _ _ _ _ _ _ _ _ _ _ _ _ _ _ _ _ _ _ _ _ _ _ _ _ _ _] -> w7
      tunnel: [w18 w357 w363 w381 w385 w403 w406 w416 w419 w425 w438 w445 w454 w481 w487 w502 w505 w525 w573 w620 w627 w670 w717 w774 w816 w863 w904 w947 w1004 w1043 w1047 w1052] -> w6
      tunnel: w4 -> [w17 _ _ _ _ _ _ _ _ _ _ _ _ _ _ _ _ _ _ _ _ _ _ _ _ _ _ _ _ _ _ _]
      tunnel: w3 -> [w15 w358 w366 w380 w395 w402 w407 w411 w421 w426 w430 w444 w456 w482 w486 w492 w506 w518 w537 w583 w630 w672 w712 w740 w785 w819 w866 w946 w983 w1018 w1046 w1051]
      frame "", "Event Structure", "Idle" {
        # "executes when the state queue is empty"
        n5 = event shown="[6] \"PS Heat\": Value Change" {
          selector: _ -> [_ _ _ _ _ _ _ _ _ _ _ _ _]
          dyn-events: _ -> [_ _ _ _ _ _ _ _ _ _ _ _ _]
          timeout: w17 -> [_ _ _ _ _ _ _ _ _ _ _ _ _]
          tunnel: w20 -> [w45 w87 w98 w120 w141 w164 w190 w254 w285 w326 w329 w350 w356]
          tunnel: [w44 w87 w98 w120 w141 w164 w190 w254 w285 w326 w329 w349 w355] -> w19
          tunnel: [w39 w86 w99 w121 w142 w163 w191 w250 w284 w318 w344 w347 w353] -> w18
          tunnel: w16 -> [w40 w86 w99 w121 w142 w163 w191 w250 w284 w318 w344 w347 w353]
          tunnel: w15 -> [w23 w89 w95 w116 w136 w158 w184 w253 w282 w323 w331 w348 w354]
          tunnel: [w33 w88 w97 w113 w143 w165 w189 w251 w281 w306 w332 w348 w354] -> w14
          event Timeout {
            n6 = event-data() -> ()  [unwired: 1 in, 1 out]
            n7 = Unbundle By Name(w40) -> ("sentinel"=w42:bool)
            n8 = call "FGV_PSP - Mercury Remote.vi"("error in"=w23, "Function"=enum16{"write", "read"}."read") -> ("error out"=w22:errorcluster, "Mercury Remote"=w21:bool)  [unwired: 4 in]
            n9 = Not(x=w42) -> (.not. x?=w41:bool)
            "Sentinel" <- w41
            n10 = Bundle(cluster=T35 {"Hold"=FALSE, "Clamp"=FALSE, "To Set"=FALSE, "To Zero"=FALSE, "Send to IPS"=FALSE, "PS Heat"=FALSE, "Lambda"=FALSE}, "Hold"="Hold", "Clamp"="Clamp", "To Set"="To Set", "To Zero"="To Zero", "Send to IPS"="Send to IPS", "PS Heat"="PS Heat", "Lambda"="Lambda") -> (w31:T35)
            n11 = local write "Remote Mode"(w21) -> ()
            n12 = case shown="True" "Lambda" {
              frame False {
                n13 = local write "LPF on (s)"(0 ("LPF on (s)")) -> ()
              }
              frame True {
                n14 = local read "LPF ON"() -> (w49:timestamp)
                n15 = Get Date/Time In Seconds() -> (seconds since 1Jan1904=w48:timestamp)
                n16 = Subtract(x=w48, y=w49) -> (x-y=→"LPF on (s)":dbl)
              }
            }
            n17 = Bundle By Name(cluster=w40, "sentinel"=w41) -> (w39:T47)
            n18 = case shown="False" w21 {
              tunnel: [w50 w76] -> w32
              tunnel: w22 -> [w50 w75]
              tunnel: w31 -> [w51 w74]
              tunnel: [w51 w66] -> w30
              frame False {
              }
              frame True {
                n19 = call "FGV_PSP - Mercury Actions.vi"("error in"=w75, "Function"=enum16{"write", "read"}."read", "mercury actions"=w74) -> ("error out"=w76:errorcluster, "mercury actions 2"=w66:T35)  [unwired: 3 in]
                n20 = Unbundle By Name(w66) -> ("Hold"=w58:bool, "Clamp"=w60:bool, "To Set"=w61:bool, "To Zero"=w62:bool, "PS Heat"=w63:bool, "Lambda"=w64:bool, "Send to IPS"=w65:bool)
                n21 = local read "Send to IPS"() -> (w59:bool)
                n22 = local read "Lambda"() -> (w57:bool)
                n23 = local read "PS Heat"() -> (w56:bool)
                n24 = local read "To Zero"() -> (w55:bool)
                n25 = local read "Clamp"() -> (w53:bool)
                n26 = local read "Hold"() -> (w52:bool)
                n27 = local read "To Set"() -> (w54:bool)
                n28 = Not Equal?(x=w59, y=w65) -> (x != y?=w67:bool)
                n29 = Not Equal?(x=w52, y=w58) -> (x != y?=w73:bool)
                n30 = Not Equal?(x=w54, y=w61) -> (x != y?=w71:bool)
                n31 = Not Equal?(x=w55, y=w62) -> (x != y?=w70:bool)
                n32 = Not Equal?(x=w56, y=w63) -> (x != y?=w69:bool)
                n33 = Not Equal?(x=w53, y=w60) -> (x != y?=w72:bool)
                n34 = Not Equal?(x=w57, y=w64) -> (x != y?=w68:bool)
                n35 = case shown="True" w73 {
                  tunnel: w58 -> [_ w84]
                  frame False {
                  }
                  frame True {
                    n36 = property on="Hold" class="Bool (strict)"("Val(Sgnl)"=w84) -> ()  [unwired: 2 in, 2 out]
                  }
                }
                n37 = case shown="True" w72 {
                  tunnel: w60 -> [_ w83]
                  frame False {
                  }
                  frame True {
                    n38 = property on="Clamp" class="Bool (strict)"("Val(Sgnl)"=w83) -> ()  [unwired: 2 in, 2 out]
                  }
                }
                n39 = case shown="True" w71 {
                  tunnel: w61 -> [_ w82]
                  frame False {
                  }
                  frame True {
                    n40 = property on="To Set" class="Bool (strict)"("Val(Sgnl)"=w82) -> ()  [unwired: 2 in, 2 out]
                  }
                }
                n41 = case shown="True" w70 {
                  tunnel: w62 -> [_ w81]
                  frame False {
                  }
                  frame True {
                    n42 = property on="To Zero" class="Bool (strict)"("Val(Sgnl)"=w81) -> ()  [unwired: 2 in, 2 out]
                  }
                }
                n43 = case shown="True" w69 {
                  tunnel: w63 -> [_ w80]
                  frame False {
                  }
                  frame True {
                    n44 = property on="PS Heat" class="Bool (strict)"("Val(Sgnl)"=w80) -> ()  [unwired: 2 in, 2 out]
                  }
                }
                n45 = case shown="True" w68 {
                  tunnel: w64 -> [_ w79]
                  frame False {
                  }
                  frame True {
                    n46 = property on="Lambda" class="Bool (strict)"("Val(Sgnl)"=w79) -> ()  [unwired: 2 in, 2 out]
                  }
                }
                n47 = case shown="True" w67 {
                  tunnel: w65 -> [_ w78]
                  frame False {
                  }
                  frame True {
                    n48 = property on="Send to IPS" class="Bool (strict)"("Val(Sgnl)"=w78) -> ()  [unwired: 2 in, 2 out]
                  }
                }
              }
            }
            n49 = call "FGV_PSP - Mercury Actions.vi"("error in"=w32, "Function"=enum16{"write", "read"}."write", "mercury actions"=w30) -> ("error out"=w33:errorcluster)  [unwired: 3 in, 1 out]
            n50 = Wait Until Next ms Multiple(millisecond multiple=u32 0) -> ()  [unwired: 1 out]
            n51 = call <vilib>:"Add State(s) to Queue__JKI_lib_State_Machine.vi"("State(s) in (\"\")"=w45, "State(s) at Back (\"\")"="#Mercury: Query ITC: Temperature\n#Mercury: Query ITC: Heater\n#Mercury: Query ITC: Aux\n#Mercury: Query ITC: Pressure\n#Mercury: Query IPS: System\n#Mercury: Query IPS: LVL\n#Mercury: Query IPS: Temperature\n#Mercury: Query IPS: Magnet\nMercury: IPS: Idle - 1\nMercury: IPS: Idle - 2\nMercury: IPS: Idle - 3\nMercury: ITC: Idle" ("State(s) at Back (\"\")")) -> ("States Out"=w44:string)  [unwired: 13 in]
          }
          event "Remote Mode": Value Change {
            n52 = event-data() -> ()  [unwired: 1 in, 6 out]
            n53 = local read "Remote Mode"() -> (w85:bool)
            n54 = call "FGV_PSP - Mercury Remote.vi"("error in"=w89, "Function"=enum16{"write", "read"}."write", "Mercury Remote"=w85) -> ("error out"=w88:errorcluster)  [unwired: 3 in, 1 out]
          }
          event "Hold": Value Change {
            n55 = event-data() -> ()  [unwired: 1 in, 6 out]
            n56 = Unbundle By Name(w99) -> ("Mercury IPS Ref"=w93:T46)
            n57 = local read "Device Identifier"() -> (w94:T33)
            n58 = local read "Hold"() -> (w91:bool)
            n59 = call-poly <instrlib>:"Open.vi"("error in (no error)"=w95, "Device Identifier"=w94, "Mercury Reference In"=w93) -> ("error out"=w96:errorcluster, "Mercury Reference Out"=w92:T46)  [unwired: 7 out]
            n60 = case shown="True" w91 {
              tunnel: [w100 w102] -> w97
              tunnel: w96 -> [w100 w111]
              tunnel: w92 -> [_ w110]
              frame False {
              }
              frame True {
                w107 = FALSE ("Hold")
                n61 = call-poly <instrlib>:"Signals (Set).vi"("error in"=w111, "PSU Act Stat"=T36 "HOLD", "Mercury Reference In"=w110) -> ("error out"=w101:errorcluster, "Response"=w109:T48)  [unwired: 1 in, 6 out]
                n62 = call "FGV_PSP - Mercury Actions.vi"("error in"=w101, "Function"=enum16{"write", "read"}."read") -> ("error out"=w104:errorcluster, "mercury actions 2"=w108:T35)  [unwired: 4 in]
                n63 = local write "Hold"(w107) -> ()
                n64 = local write "Magnet Status 2"(w109) -> ()
                n65 = Bundle By Name(cluster=w108, "Hold"=w107) -> (w106:T35)
                n66 = call "FGV_PSP - Mercury Actions.vi"("error in"=w104, "Function"=enum16{"write", "read"}."write", "mercury actions"=w106) -> ("error out"=w102:errorcluster)  [unwired: 3 in, 1 out]
              }
            }
          }
          event "Clamp": Value Change {
            n67 = event-data() -> ()  [unwired: 1 in, 6 out]
            n68 = Unbundle By Name(w121) -> ("Mercury IPS Ref"=w115:T46)
            n69 = local read "Device Identifier"() -> (w119:T33)
            n70 = local read "Clamp"() -> (w114:bool)
            n71 = call-poly <instrlib>:"Open.vi"("error in (no error)"=w116, "Device Identifier"=w119, "Mercury Reference In"=w115) -> ("error out"=w118:errorcluster, "Mercury Reference Out"=w117:T46)  [unwired: 7 out]
            n72 = case shown="True" w114 {
              tunnel: w118 -> [w122 w132]
              tunnel: w117 -> [_ w131]
              tunnel: [w122 w124] -> w113
              frame False {
              }
              frame True {
                w123 = FALSE
                n73 = call-poly <instrlib>:"Signals (Set).vi"("error in"=w132, "PSU Act Stat"=T36 "CLMP", "Mercury Reference In"=w131) -> ("error out"=w125:errorcluster, "Response"=w133:T48)  [unwired: 1 in, 6 out]
                n74 = call "FGV_PSP - Mercury Actions.vi"("error in"=w125, "Function"=enum16{"write", "read"}."read") -> ("error out"=w127:errorcluster, "mercury actions 2"=w130:T35)  [unwired: 4 in]
                n75 = local write "Clamp"(w123) -> ()
                n76 = Bundle By Name(cluster=w130, "Clamp"=w123) -> (w129:T35)
                n77 = local write "Magnet Status 2"(w133) -> ()
                n78 = call "FGV_PSP - Mercury Actions.vi"("error in"=w127, "Function"=enum16{"write", "read"}."write", "mercury actions"=w129) -> ("error out"=w124:errorcluster)  [unwired: 3 in, 1 out]
              }
            }
          }
          event "To Set": Value Change {
            n79 = event-data() -> ()  [unwired: 1 in, 6 out]
            n80 = Unbundle By Name(w142) -> ("Mercury IPS Ref"=w138:T46)
            n81 = local read "Device Identifier"() -> (w137:T33)
            n82 = call-poly <instrlib>:"Open.vi"("error in (no error)"=w136, "Device Identifier"=w137, "Mercury Reference In"=w138) -> ("error out"=w139:errorcluster, "Mercury Reference Out"=w140:T46)  [unwired: 7 out]
            n83 = local read "To Set"() -> (w135:bool)
            n84 = case shown="True" w135 {
              tunnel: [w144 w146] -> w143
              tunnel: w140 -> [_ w154]
              tunnel: w139 -> [w144 w153]
              frame False {
              }
              frame True {
                w145 = FALSE
                n85 = call-poly <instrlib>:"Signals (Set).vi"("error in"=w153, "PSU Act Stat"=T36 "RTOS", "Mercury Reference In"=w154) -> ("error out"=w147:errorcluster, "Response"=w155:T48)  [unwired: 1 in, 6 out]
                n86 = call "FGV_PSP - Mercury Actions.vi"("error in"=w147, "Function"=enum16{"write", "read"}."read") -> ("error out"=w149:errorcluster, "mercury actions 2"=w152:T35)  [unwired: 4 in]
                n87 = Bundle By Name(cluster=w152, "To Set"=w145) -> (w151:T35)
                n88 = local write "To Set"(w145) -> ()
                n89 = local write "Magnet Status 2"(w155) -> ()
                n90 = call "FGV_PSP - Mercury Actions.vi"("error in"=w149, "Function"=enum16{"write", "read"}."write", "mercury actions"=w151) -> ("error out"=w146:errorcluster)  [unwired: 3 in, 1 out]
              }
            }
          }
          event "To Zero": Value Change {
            n91 = event-data() -> ()  [unwired: 1 in, 6 out]
            n92 = Unbundle By Name(w163) -> ("Mercury IPS Ref"=w160:T46)
            n93 = local read "Device Identifier"() -> (w159:T33)
            n94 = local read "To Zero"() -> (w157:bool)
            n95 = call-poly <instrlib>:"Open.vi"("error in (no error)"=w158, "Device Identifier"=w159, "Mercury Reference In"=w160) -> ("error out"=w161:errorcluster, "Mercury Reference Out"=w162:T46)  [unwired: 7 out]
            n96 = case shown="True" w157 {
              tunnel: [w166 w169] -> w165
              tunnel: w162 -> [_ w176]
              tunnel: w161 -> [w166 w175]
              frame False {
              }
              frame True {
                w167 = FALSE
                n97 = call-poly <instrlib>:"Signals (Set).vi"("error in"=w175, "PSU Act Stat"=T36 "RTOZ", "Mercury Reference In"=w176) -> ("error out"=w170:errorcluster, "Response"=w177:T48)  [unwired: 1 in, 6 out]
                n98 = call "FGV_PSP - Mercury Actions.vi"("error in"=w170, "Function"=enum16{"write", "read"}."read") -> ("error out"=w172:errorcluster, "mercury actions 2"=w168:T35)  [unwired: 4 in]
                n99 = Bundle By Name(cluster=w168, "To Zero"=w167) -> (w174:T35)
                n100 = local write "To Zero"(w167) -> ()
                n101 = local write "Magnet Status 2"(w177) -> ()
                n102 = call "FGV_PSP - Mercury Actions.vi"("error in"=w172, "Function"=enum16{"write", "read"}."write", "mercury actions"=w174) -> ("error out"=w169:errorcluster)  [unwired: 3 in, 1 out]
              }
            }
          }
          event "PS Heat": Value Change {
            n103 = event-data() -> ()  [unwired: 1 in, 6 out]
            n104 = local read "Device Identifier"() -> (w185:T33)
            n105 = Unbundle By Name(w191) -> ("Mercury IPS Ref"=w187:T46)
            n106 = call-poly <instrlib>:"Open.vi"("error in (no error)"=w184, "Device Identifier"=w185, "Mercury Reference In"=w187) -> ("error out"=w181:errorcluster, "Mercury Reference Out"=w182:T46)  [unwired: 7 out]
            n107 = call-poly <instrlib>:"Signals (Read).vi"("error in"=w181, "Mercury Reference In"=w182) -> ("error out"=w193:errorcluster, "Current"=w188:dbl, "Mercury Reference Out"=w192:T46)  [unwired: 1 in, 6 out]
            n108 = local read "PS Heat"() -> (w180:bool)
            n109 = call-poly <instrlib>:"Signals (Read).vi"("error in"=w193, "Mercury Reference In"=w192) -> ("error out"=w194:errorcluster, "Persistant Current"=w183:dbl, "Mercury Reference Out"=w195:T46)  [unwired: 1 in, 6 out]
            n110 = Subtract(x=w183, y=w188) -> (x-y=w196:dbl)
            n111 = Absolute Value(x=w196) -> (abs(x)=w197:dbl)
            n112 = Less?(x=w197, y=0.1) -> (x < y?=w199:bool)
            n113 = case shown="False" w199 {
              selector: w199 -> [_ w202]
              tunnel: [w201 w202] -> w179
              frame False {
                n114 = Two Button Dialog(message="The magnet current is more\nthan 0.1A different to the\nPSU output current.  It is not\nadvisable to switch on the\nswitch heater unless these\ncurrents are equal!") -> (T button?=w201:bool)  [unwired: 2 out]
              }
              frame True {
              }
            }
            n115 = And(x=w180, y=w179) -> (x .and. y?=w186:bool)
            n116 = case shown="True" w186 {
              tunnel: w195 -> [_ w213]
              tunnel: w194 -> [w203 w212]
              tunnel: [w203 w204] -> w189
              frame False {
              }
              frame True {
                w206 = FALSE
                n117 = flat-sequence {
                  tunnel: [w224] -> w221
                  tunnel: [w223] -> w220
                  tunnel: [w222] -> w219
                  tunnel: w213 -> [w226]
                  tunnel: w212 -> [w225]
                  tunnel: w221 -> [w229]
                  tunnel: w220 -> [w228]
                  tunnel: [w229] -> w218
                  tunnel: [w228] -> w217
                  tunnel: [w227] -> w216
                  tunnel: w219 -> [w227]
                  tunnel: w218 -> [w240]
                  tunnel: w217 -> [w241]
                  tunnel: w216 -> [w238]
                  tunnel: [w235] -> w215
                  tunnel: [w236] -> w214
                  tunnel: w215 -> [w245]
                  tunnel: w214 -> [w244]
                  tunnel: [w243] -> w205
                  frame #0 {
                    n118 = call-poly <instrlib>:"Signals (Read).vi"("error in"=w225, "Mercury Reference In"=w226) -> ("error out"=w224:errorcluster, "Switch Heater Status"=w222:string, "Mercury Reference Out"=w223:T46)  [unwired: 1 in, 6 out]
                  }
                  frame #1 {
                    n119 = Wait Until Next ms Multiple(millisecond multiple=u32 100) -> ()  [unwired: 1 out]
                  }
                  frame #2 {
                    n120 = Equal?(x=w238, y="ON") -> (x = y?=w237:bool)
                    n121 = Select(t=T37 "OFF" ("Set Switch Heater"), s=w237, f=T37 "ON" ("Set Switch Heater")) -> (s? t:f=w232:T37)
                    n122 = call-poly <instrlib>:"Signals (Set).vi"("error in"=w240, "Set Switch Heater"=w232, "Mercury Reference In"=w241) -> ("error out"=w236:errorcluster, "Response"=w231:T48, "Mercury Reference Out"=w235:T46)  [unwired: 1 in, 5 out]
                    n123 = local write "Magnet Status 2"(w231) -> ()
                  }
                  frame #3 {
                    n124 = call-poly <instrlib>:"Configuration (Read).vi"("error in"=w244, "Mercury Reference In"=w245) -> ("error out"=w243:errorcluster, "Time"=→"Switch Time":string)  [unwired: 1 in, 7 out]
                  }
                }
                n125 = call "FGV_PSP - Mercury Actions.vi"("error in"=w205, "Function"=enum16{"write", "read"}."read") -> ("error out"=w209:errorcluster, "mercury actions 2"=w207:T35)  [unwired: 4 in]
                n126 = local write "PS Heat"(w206) -> ()
                n127 = Bundle By Name(cluster=w207, "PS Heat"=w206) -> (w211:T35)
                n128 = call "FGV_PSP - Mercury Actions.vi"("error in"=w209, "Function"=enum16{"write", "read"}."write", "mercury actions"=w211) -> ("error out"=w204:errorcluster)  [unwired: 3 in, 1 out]
              }
            }
          }
          event "Send to IPS": Value Change {
            n129 = event-data() -> ()  [unwired: 1 in, 6 out]
            n130 = local read "Device Identifier"() -> (w249:T33)
            n131 = Unbundle By Name(w250) -> ("Mercury IPS Ref"=w248:T46)
            n132 = local read "Send to IPS"() -> (w246:bool)
            n133 = call-poly <instrlib>:"Open.vi"("error in (no error)"=w253, "Device Identifier"=w249, "Mercury Reference In"=w248) -> ("error out"=w252:errorcluster, "Mercury Reference Out"=w247:T46)  [unwired: 7 out]
            n134 = case shown="True" w246 {
              tunnel: w252 -> [w255 w274]
              tunnel: [w255 w258] -> w251
              tunnel: w247 -> [_ w272]
              frame False {
              }
              frame True {
                w257 = FALSE
                n135 = local read "Remote Mode"() -> (w270:bool)
                n136 = case shown="True" w270 {
                  tunnel: "Target Field (T)" -> [w276 _]
                  tunnel: "Target Rate (T/min)" -> [w275 _]
                  tunnel: [w276 w278] -> w264
                  tunnel: [w275 w277] -> w265
                  frame False {
                  }
                  frame True {
                    n137 = call "FGV_PSP - Mercury Targets.vi"("Function"=enum16{"write", "read"}."read") -> ("Mercury Targets"=w279:T49)  [unwired: 5 in, 1 out]
                    n138 = Unbundle(w279) -> ("Target Field (T)"=w278:dbl, "Target Field Rate (T/min)"=w277:dbl)
                  }
                }
                n139 = local write "Send to IPS"(w257) -> ()
                n140 = call-poly <instrlib>:"Signals (Set).vi"("error in"=w274, "Target Field Rate"=w265, "Mercury Reference In"=w272) -> ("error out"=w273:errorcluster, "Mercury Reference Out"=w271:T46)  [unwired: 2 in, 5 out]
                n141 = local write "Target Field (T)"(w264) -> ()
                n142 = local write "Target Rate (T/min)"(w265) -> ()
                n143 = Bundle("Target Field (T)"=w264, "Target Field Rate (T/min)"=w265) -> (w267:T49)  [unwired: 1 in]
                n144 = call-poly <instrlib>:"Signals (Set).vi"("error in"=w273, "Target Field"=w264, "Mercury Reference In"=w271) -> ("error out"=w256:errorcluster)  [unwired: 2 in, 6 out]
                n145 = call "FGV_PSP - Mercury Actions.vi"("error in"=w256, "Function"=enum16{"write", "read"}."read") -> ("error out"=w261:errorcluster, "mercury actions 2"=w259:T35)  [unwired: 4 in]
                n146 = Bundle By Name(cluster=w259, "Send to IPS"=w257) -> (w263:T35)
                n147 = call "FGV_PSP - Mercury Actions.vi"("error in"=w261, "Function"=enum16{"write", "read"}."write", "mercury actions"=w263) -> ("error out"=w258:errorcluster)  [unwired: 3 in, 1 out]
                n148 = call "FGV_PSP - Mercury Targets.vi"("Function"=enum16{"write", "read"}."write", "Mercury Targets"=w267) -> ()  [unwired: 4 in, 2 out]
              }
            }
          }
          event "Lambda": Value Change {
            n149 = event-data() -> ()  [unwired: 1 in, 6 out]
            n150 = Unbundle By Name(w284) -> ("Mercury ITC Ref"=w283:T50)
            n151 = disable-structure shown="Disabled" {
              disable-tunnel: w283 -> [w302 _]
              disable-tunnel: w282 -> [w299 _]
              disable-tunnel: [w287 _] -> w281
              frame Disabled {
                # "TEMP device"
                # "AUX\nPRES\nHTR\nTEMP"
                n152 = local read "ITC Devices"() -> (w303:string[])
                n153 = Index Array(array=w303, index=3 ("Lambda device")) -> (element=w301:string)
                n154 = call-poly <instrlib>:"Open.vi"("error in (no error)"=w299, "Device Identifier"=w301, "Mercury Reference In"=w302) -> ("error out"=w291:errorcluster, "Mercury Reference Out"=w290:T46)  [unwired: 1 in, 6 out]
                n155 = local read "Lambda"() -> (w298:bool)
                n156 = call <instrlib>:"Build SCPI Command.vi"("error in"=w291, "Noun(s)"=":SIG:PERC:", "Verb"=T38 "SET:", "Mercury Reference In"=w290) -> ("error out"=w288:errorcluster, "SCPI Message(s)"=w292:string[], "Mercury Reference Out"=w294:T46)  [unwired: 5 in]
                n157 = Select(t="ON" ("Sweep Mode"), s=w298, f="OFF" ("Sweep Mode")) -> ()  [unwired: 1 out]
                n158 = case shown="True" w298 {
                  frame False {
                    n159 = local write "LPF ON"(timestamp(0 s since 1904-01-01) ("LPF ON")) -> ()
                  }
                  frame True {
                    n160 = Get Date/Time In Seconds() -> (seconds since 1Jan1904=w305:timestamp)
                    n161 = local write "LPF ON"(w305) -> ()
                  }
                }
                n162 = call <instrlib>:"Set (Str).vi"("ISOBUS address"=T39 -1, "error in"=w288, "SCPI Message(s)"=w292, "Mercury Reference In"=w294) -> ("error out"=w287:errorcluster, "Response"=w286:T48)  [unwired: 4 in, 2 out]
                n163 = local write "Magnet Status 2"(w286) -> ()
              }
              frame Enabled {
              }
            }
          }
          event "Fast/Slow Fill": Value Change {
            n164 = event-data() -> ()  [unwired: 1 in, 6 out]
            n165 = local read "IPS Devices"() -> (w320:string[])
            n166 = Unbundle By Name(w318) -> ("Mercury IPS Ref"=w325:T46)
            n167 = Index Array(array=w320, index=0) -> (element=w319:string)
            n168 = call-poly <instrlib>:"Open.vi"("error in (no error)"=w323, "Device Identifier"=w319, "Mercury Reference In"=w325) -> ("error out"=w316:errorcluster, "Mercury Reference Out"=w324:T46)  [unwired: 7 out]
            n169 = local read "Fast/Slow Fill"() -> (w311:bool)
            n170 = call <instrlib>:"Build SCPI Command.vi"("error in"=w316, "Noun(s)"=":HEL:PULS:SLOW:", "Verb"=T38 "SET:", "Mercury Reference In"=w324) -> ("error out"=w309:errorcluster, "SCPI Message(s)"=w314:string[], "Mercury Reference Out"=w308:T46)  [unwired: 5 in]
            n171 = Select(t="OFF" ("Temperature setpoint"), s=w311, f="ON" ("Temperature setpoint")) -> (s? t:f=w313:string)
            n172 = call <instrlib>:"Set (Str).vi"("ISOBUS address"=T39 -1, "error in"=w309, "Command Value (Str)"=w313, "SCPI Message(s)"=w314, "Mercury Reference In"=w308) -> ("error out"=w306:errorcluster, "Response"=w307:T48)  [unwired: 5 out]
            n173 = local write "Magnet Status 2"(w307) -> ()
          }
          event "Set Needle Valve (%)": Value Change {
            n174 = event-data() -> ("NewVal"=w333:dbl)  [unwired: 1 in, 5 out]
            n175 = Unbundle By Name(w344) -> ("Mercury ITC Ref"=w345:T50)
            n176 = local read "ITC Devices"() -> (w342:string[])
            n177 = Index Array(array=w342, index=3) -> (element=w341:string)
            n178 = call-poly <instrlib>:"Open.vi"("error in (no error)"=w331, "Device Identifier"=w341, "Mercury Reference In"=w345) -> ("error out"=w335:errorcluster, "Mercury Reference Out"=w334:T46)  [unwired: 7 out]
            n179 = call <instrlib>:"Build SCPI Command.vi"("error in"=w335, "Noun(s)"=":LOOP:FSET:", "Verb"=T38 "SET:", "Mercury Reference In"=w334) -> ("error out"=w336:errorcluster, "SCPI Message(s)"=w327:string[], "Mercury Reference Out"=w338:T46)  [unwired: 5 in]
            n180 = call <instrlib>:"Set (DBL).vi"("ISOBUS address"=T39 -1, "Unit"=T3 "", "error in"=w336, "Command Value (Dbl)"=w333, "SCPI Message(s)"=w327, "Mercury Reference In"=w338) -> ("error out"=w332:errorcluster, "Response"=w328:T48)  [unwired: 2 in, 2 out]
            n181 = local write "Magnet Status 2"(w328) -> ()
          }
          event "OK": Value Change {
            # "Exit Button Value Change (pressed) Event\n(this executes Macro: Exit to terminate the VI)"
            n182 = event-data() -> ()  [unwired: 1 in, 1 out]
            n183 = call <vilib>:"Add State(s) to Queue__JKI_lib_State_Machine.vi"("State(s) in Front (\"\")"="Macro: Exit", "State(s) in (\"\")"=w350) -> ("States Out"=w349:string)  [unwired: 13 in]
          }
          event Panel Close? {
            # "Discard the event because we'll close the front panel ourselves in Macro: Exit"
            # "Close Panel button (pressed) Event\n(this executes Macro: Exit to terminate the VI)"
            n184 = event-data() -> ()  [unwired: 1 in, 1 out]
            n185 = call <vilib>:"Add State(s) to Queue__JKI_lib_State_Machine.vi"("State(s) in Front (\"\")"="Macro: Exit", "State(s) in (\"\")"=w356) -> ("States Out"=w355:string)  [unwired: 13 in]
            n186 = event-data("Discard?"=TRUE) -> ()  [unwired: 1 in, 1 out]
          }
        }
      }
      frame "---------- Core ----------" {
        # "Do not put any code in this frame.\n(it is a separator no-op)"
        n187 = call <vilib>:"Add State(s) to Queue__JKI_lib_State_Machine.vi"("State(s) in (\"\")"=w360) -> ("States Out"=w359:string)  [unwired: 14 in]
      }
      frame Default {
        w370 = 42 items=["No error", "Argument error", "Memory is full", "Out of zone", "End of file", "File already open", "Generic file I/O error", "File not found", "File permission error", "Disk is full", "Duplicate path", "Too many files open", "System feature not enabled", "Resource file not found", "Cannot add resource", "Resource not found", "Image not found", "Image memory error", "Pen does not exist", "Config type invalid", "Config token not found", "Config parse error", "Config memory error", "Bad external code format", "Bad external code offset", "External code not present", "Null window", "Destroy window error", "Null menu", "Print aborted", "Bad print record", "Print driver error", "Windows error during printing", "Memory error during printing", "Print dialog error", "Generic print error", "Invalid device refnum", "Device not found", "Device parameter error", "Device unit error", "Cannot open device", "Device call aborted", "Generic error", "Cancelled by user", "Object ID too low", "Object ID too high", "Object not in heap", "Unknown heap", "Unknown object (invalid DefProc)", "Unknown object (DefProc not in table)", "Message out of range", "Invalid (null) method", "Unknown message", "Manager call not supported", "Bad address", "Network operation in progress", "Network operation timed out", "Connection is busy", "Network attribute not supported", "Network error", "Address in use", "System out of memory", "Connection aborted", "Connection refused", "Not connected", "Already connected", "Connection closed", "Initialization error (interapplication manager)", "Bad occurrence", "Wait on unbound occurrence handler", "Occurrence queue overflow", "Datalog type conflict", "Unused", "Unrecognized type (interapplication manager)", "Memory corrupt", "Failed to make temporary DLL", "Old CIN version", "Drag socket not found", "Failed to load drop-object", "Failed to register OLE object", "Failed to release OLE object", "Format specifier type mismatch", "Unknown format specifier", "Too few format specifiers", "Too many format specifiers", "Scan failed", "Newer CIN version", "Error converting to variant", "Runtime menu error", "Password tampered", "Variant attribute not found", "Incompatible variant data type", "Event data is not available", "Event Store is not present", "Occurrence is not found", "Event Queue is not created", "Event info is not available", "Refnum passed is NULL", "Error retrieving Class GUID", "Error retrieving CoClass GUID", "Error retrieving TypeLib GUID.", "Bad built application magic bytes.", "Specific driver is different from the specific driver associated with the Logical Name.", "There is no session opened to the class driver.", "Max Error", "MAX - Error with config objects", "MAX - Error loading configuration", "MAX - Group not supported"]
        # "Current State"
        # "Do not delete, rename, or modify this frame.\n(this is used to capture unhandled states and typos)"
        # "Handle mistyped state name (developer tool)"
        n188 = Format Into String(format string="Software Exception: Unhandled State \"%s\"." ("message"), error in=w366, w361) -> (resulting string=w369:string, error out=w368:errorcluster)  [unwired: 1 in]
        n189 = call <vilib>:"Error Cluster From Error Code.vi"("show call chain? (False)"=TRUE, "error in (no error)"=w368, "error message (\"\")"=w369, "error code (0)"=w370) -> ("error out"=w367:errorcluster)  [unwired: 5 in]
        n190 = call <vilib>:"Add State(s) to Queue__JKI_lib_State_Machine.vi"("State(s) in (\"\")"=w365) -> ("States Out"=w364:string)  [unwired: 14 in]
      }
      frame "Initialize Core Data" {
        # "Do not delete, rename, or modify this frame.\n(this is used to determine panel behavior on exit)"
        # "originally closed?"
        # "exe?"
        # "If panel starts closed or is an EXE, then close it when we exit"
        n191 = property class="VI"() -> ("Front Panel.Open"=w379:bool)  [unwired: 2 in, 2 out]
        n192 = property class="App"() -> ("App.Kind"=w378:T40)  [unwired: 2 in, 2 out]
        n193 = control-ref of="Current VI Reference"() -> (w372:refnum<vi>)
        n194 = Not(x=w379) -> (.not. x?=w376:bool)
        n195 = Equal?(x=w378, y=T40."Run Time System" ("Application:Kind")) -> (x = y?=w375:bool)
        n196 = Or(x=w376, y=w375) -> (x .or. y?=w373:bool)
        n197 = Bundle By Name(cluster=w374, "Core.Current VI Reference"=w372, "Core.Close Panel on Exit?"=w373) -> (w381:T47)
        n198 = call <vilib>:"Add State(s) to Queue__JKI_lib_State_Machine.vi"("State(s) in (\"\")"=w383) -> ("States Out"=w382:string)  [unwired: 14 in]
      }
      frame "Error Handler" {
        w394 = i32[] [-1950679035, -1950678943]  # Error Codes to Filter
        # "Unhandled Error -- Display it"
        # "Handle any errors here.\nYou can also output any states to clean-up after errors occur"
        # "Clear error"
        n199 = call-poly <userlib>:"Filter Error Codes__ogtk.vi"("Error In"=w395, "Error Codes to Filter"=w394) -> ("Error Out"=w396:errorcluster, "Filtered Error Details"=w393:T51)  [unwired: 7 in, 1 out]
        n200 = Unbundle(w393) -> ("code"=w391:i32, "source"=w392:string)
        n201 = Get Date/Time In Seconds() -> (seconds since 1Jan1904=w390:timestamp)
        n202 = Unbundle By Name(w386) -> ("Error Log"=w388:T34)
        n203 = Bundle By Name(cluster=T41 {"time"=timestamp(0 s since 1904-01-01), "code"=0, "source"=""} ("output cluster"), "time"=w390, "code"=w391, "source"=w392) -> (w387:T41)
        n204 = Build Array (concatenate)(w388, w387) -> (w384:T34)
        "Error List" <- w384
        n205 = Bundle By Name(cluster=w386, "Error Log"=w384) -> (w385:T47)
        n206 = call <vilib>:"General Error Handler.vi"("error in (no error)"=w396) -> ()  [unwired: 10 in, 5 out]
        n207 = call <vilib>:"Add State(s) to Queue__JKI_lib_State_Machine.vi"("State(s) in Front (\"\")"="/* Post Error States", "State(s) in (\"\")"=w400) -> ("States Out"=w399:string)  [unwired: 13 in]
      }
      frame "Exit" {
        # "Do not put any code in this frame.\n(No errors that occur here will be handled.)"
        n208 = call <vilib>:"Add State(s) to Queue__JKI_lib_State_Machine.vi"("State(s) in (\"\")"=w405) -> ("States Out"=w404:string)  [unwired: 14 in]
      }
      frame "---------- Data ----------" {
        # "Do not put any code in this frame.\n(It is a separator no-op. You can make a copy of this frame to create a new Data frame)"
        n209 = call <vilib>:"Add State(s) to Queue__JKI_lib_State_Machine.vi"("State(s) in (\"\")"=w409) -> ("States Out"=w408:string)  [unwired: 14 in]
      }
      frame "Data: Initialize" {
        w410 = T34 []  # Error Log
        w412 = TRUE  # sentinel
        w413 = T46 {"Comms"="", "Device ID"=[], "Comms Layer"=enum."Ethernet TCP/IP", "Command"="", "Query reference"=refnum}  # Mercury IPS Ref
        w414 = T50 {"Comms"="", "Device ID"=[], "Comms Layer"=enum."Ethernet TCP/IP", "Command"="", "Query reference"=refnum}  # Mercury ITC Ref
        w415 = T52 {"Current VI Reference"=refnum, "Close Panel on Exit?"=FALSE}  # Core
        # "do not delete - used by framework"
        # "Expand Bundle to add new data elements to shift register data."
        # "Add new data here."
        # "Data names and types of shift register data are defined by this bundle."
        # "Initialize the shift-register data, here.\n(data names are defined by what you wire into the bundle function)"
        n210 = Bundle("Core"=w415, "Mercury ITC Ref"=w414, "Mercury IPS Ref"=w413, "sentinel"=w412, "Error Log"=w410) -> (w416:T47)  [unwired: 1 in]
        n211 = call <vilib>:"Add State(s) to Queue__JKI_lib_State_Machine.vi"("State(s) in (\"\")"=w418) -> ("States Out"=w417:string)  [unwired: 14 in]
      }
      frame "Data: Cleanup" {
        # "Cleanup any data and references, here.\n(this is called automatically, by the Macro: Exit)"
        n212 = Unbundle By Name(w419) -> ("Core.Current VI Reference"=w422:refnum<vi>)
        n213 = Close Reference(reference=w422, error in (no error)=w421) -> (error out=w420:errorcluster)
        n214 = call <vilib>:"Add State(s) to Queue__JKI_lib_State_Machine.vi"("State(s) in (\"\")"=w424) -> ("States Out"=w423:string)  [unwired: 14 in]
      }
      frame "---------- UI ----------" {
        # "Do not put any code in this frame.\n(It is a separator no-op. You can make a copy of this frame to create a new UI frame)"
        n215 = call <vilib>:"Add State(s) to Queue__JKI_lib_State_Machine.vi"("State(s) in (\"\")"=w428) -> ("States Out"=w427:string)  [unwired: 14 in]
      }
      frame "UI: Initialize" {
        w435 = FALSE
        # "start in local mode"
        # "Initialize the User Interface, here.\n(this is called automatically, by the Macro: Init)"
        n216 = disable-structure shown="Disabled" {
          frame Disabled {
            n217 = Open VI Reference(vi path=path "") -> ()  [unwired: 5 in, 2 out]
            n218 = call "MNK_Dashboard_v2.vi"() -> ()  [unwired: 12 in]
          }
          frame Enabled {
          }
        }
        n219 = Open Application Reference(8:w430) -> (0:w432:errorcluster, 3:w433:refnum<vi>)  [unwired: 3 in]
        n220 = property class="App"(reference=w433, error in=w432, "WebSrvr.Active"=TRUE ("Web Server:Server Active")) -> (error out=w429:errorcluster)  [unwired: 1 out]
        n221 = call <vilib>:"Add State(s) to Queue__JKI_lib_State_Machine.vi"("State(s) in (\"\")"=w440) -> ("States Out"=w439:string)  [unwired: 14 in]
        n222 = local write "Remote Mode"(w435) -> ()
        n223 = call "FGV - Attocube Remote.vi"("error in"=w429, "Function"=enum16{"write", "read"}."write", "Attocube Remote"=w435) -> ("error out"=w434:errorcluster)  [unwired: 3 in, 1 out]
        "Magnet Status 2" <- "" ("Magnet Status 2")
      }
      frame "UI: Cursor Set" {
        # "Argument"
        # "Set and Unset Cursor Busy.\n(Usage: \"UI: Cursor Set >> Busy|Idle\")"
        n224 = case shown="\"Idle\", Default" w442 {
          tunnel: w444 -> [w449 w451]
          tunnel: [w448 w450] -> w443
          frame "Idle", Default {
            n225 = call <vilib>:"Unset Busy.vi"("error in (no error)"=w449) -> ("error out"=w448:errorcluster)  [unwired: 10 in]
          }
          frame "Busy" {
            n226 = call <vilib>:"Set Busy.vi"("error in (no error)"=w451) -> ("error out"=w450:errorcluster)  [unwired: 9 in, 1 out]
          }
        }
        n227 = call <vilib>:"Add State(s) to Queue__JKI_lib_State_Machine.vi"("State(s) in (\"\")"=w447) -> ("States Out"=w446:string)  [unwired: 14 in]
      }
      frame "UI: Front Panel State" {
        # "Argument"
        # "Set Front Panel Open or Closed\n(Usage: \"UI: Front Panel State >> Open|Close\")"
        n228 = Unbundle By Name(w454) -> ("Core.Current VI Reference"=w453:refnum<vi>)
        n229 = case shown="\"Open\", Default" w452 {
          tunnel: w456 -> [w462 w475]
          tunnel: [w464 w476] -> w455
          tunnel: w453 -> [w463 w473]
          frame "Open", Default {
            n230 = property class="VI"(reference=w463, error in=w462) -> (reference out=w460:refnum<vi>, error out=w461:errorcluster, "Front Panel.Open"=w459:bool)
            n231 = case shown="True" w459 {
              tunnel: [w467 w470] -> w464
              tunnel: w461 -> [w466 w470]
              tunnel: w460 -> [w465 _]
              frame False {
                n232 = invoke class="VI" method="FP.Open"(reference=w465, error in=w466, "Activate"=TRUE, "State"=T42."Standard") -> (error out=w467:errorcluster)  [unwired: 1 in, 4 out]
              }
              frame True {
              }
            }
          }
          frame "Close" {
            n233 = property class="VI"(reference=w473, error in=w475) -> (reference out=w472:refnum<vi>, error out=w474:errorcluster, "Front Panel.Open"=w471:bool)
            n234 = case shown="True" w471 {
              tunnel: [w477 w480] -> w476
              tunnel: w474 -> [w477 w479]
              tunnel: w472 -> [_ w478]
              frame False {
              }
              frame True {
                n235 = invoke class="VI" method="FP.Close"(reference=w478, error in=w479) -> (error out=w480:errorcluster)  [unwired: 1 in, 2 out]
              }
            }
          }
        }
        n236 = call <vilib>:"Add State(s) to Queue__JKI_lib_State_Machine.vi"("State(s) in (\"\")"=w458) -> ("States Out"=w457:string)  [unwired: 14 in]
      }
      frame "---------- Macro ----------" {
        # "Do not put any code in this frame.\n(It is a separator no-op. You can make a copy of this frame to create a new Macro frame)"
        n237 = call <vilib>:"Add State(s) to Queue__JKI_lib_State_Machine.vi"("State(s) in (\"\")"=w484) -> ("States Out"=w483:string)  [unwired: 14 in]
      }
      frame "Macro: Initialize" {
        w485 = "Data: Initialize\nInitialize Core Data\nUI: Initialize\nUI: Front Panel State >> Open\nMercury: Initialize"  # Data: Initialize Initialize Core Data UI: Initialize UI: Front Panel State >> Open Mercury: Initialize
        # "Initialization Macro\n(This is called once, when the VI starts)"
        n238 = call <vilib>:"Add State(s) to Queue__JKI_lib_State_Machine.vi"("State(s) in Front (\"\")"=w485, "State(s) in (\"\")"=w489) -> ("States Out"=w488:string)  [unwired: 13 in]
      }
      frame "Macro: Exit" {
        # "Exit Macro\n(This is called once, when the VI exits)"
        n239 = Unbundle By Name(w502) -> ("Core.Close Panel on Exit?"=w501:bool, "Mercury ITC Ref"=w494:T50, "Mercury IPS Ref"=w493:T46)
        n240 = call <instrlib>:"Close.vi"("error in (no error)"=w492, "Mercury Reference"=w493) -> ("error out"=w491:errorcluster)  [unwired: 9 out]
        n241 = call <instrlib>:"Close.vi"("error in (no error)"=w491, "Mercury Reference"=w494) -> ("error out"=w495:errorcluster)  [unwired: 9 out]
        n242 = call <vilib>:"Simple Error Handler.vi"("error in (no error)"=w495) -> ("error out"=w490:errorcluster)  [unwired: 1 in, 7 out]
        n243 = Select(t="UI: Front Panel State >> Close", s=w501, f="") -> (s? t:f=w498:string)
        n244 = call <vilib>:"Add State(s) to Queue__JKI_lib_State_Machine.vi"("State(s) in (\"\")"=w498, "State(s) at Back (\"\")"="Data: Cleanup\nExit") -> ("States Out"=w496:string)  [unwired: 13 in]
        n245 = call <vilib>:"Add State(s) to Queue__JKI_lib_State_Machine.vi"("State(s) in Front (\"\")"=w496, "State(s) in (\"\")"=w504) -> ("States Out"=w503:string)  [unwired: 13 in]
      }
      frame "---------- New Category ----------" {
        n246 = call <vilib>:"Add State(s) to Queue__JKI_lib_State_Machine.vi"("State(s) in (\"\")"=w508) -> ("States Out"=w507:string)  [unwired: 14 in]
      }
      frame "Mercury: Initialize" {
        w517 = Comms_Transport_Layer."Ethernet TCP/IP" ("Comms Layer")
        n247 = call-poly <instrlib>:"Open.vi"("Clear Previous Connections (False)"=TRUE ("Clear Previous Connections (True)"), "ID Query (True)"=TRUE, "IP Address"="ITC IP Address", "error in (no error)"=w518, "Comms Layer"=w517) -> ("error out"=w511:errorcluster, "# of Instruments"=→"# of Instruments":i32, "Serial Number(s)"=→"Serial Number(s)":string[], "Mercury Reference Out"=w512:T46, "S/W Version(s)"=→"S/W Version(s)":string[])  [unwired: 2 in]
        n248 = call-poly <instrlib>:"Open.vi"("Clear Previous Connections (False)"=FALSE ("Clear Previous Connections (True)"), "ID Query (True)"=TRUE, "IP Address"="IPS IP Address", "error in (no error)"=w511, "Comms Layer"=w517) -> ("error out"=w510:errorcluster, "# of Instruments"=→"# of Instruments 2":i32, "Serial Number(s)"=→"Serial Number(s) 2":string[], "Mercury Reference Out"=w509:T46, "S/W Version(s)"=→"S/W Version(s) 2":string[])  [unwired: 2 in]
        n249 = Bundle By Name(cluster=w526, "Mercury ITC Ref"=w512, "Mercury IPS Ref"=w509) -> (w525:T47)
        n250 = call <vilib>:"Add State(s) to Queue__JKI_lib_State_Machine.vi"("State(s) in (\"\")"=w531, "State(s) at Back (\"\")"="Mercury: Query ITC: System\nMercury: Query IPS: System\nMercury: Query ITC: Temperature\nMercury: Query ITC: Heater\nMercury: Query ITC: Aux\nMercury: Query ITC: Pressure\nMercury: Query IPS: LVL\nMercury: Query IPS: Temperature\nMercury: Query IPS: Magnet" ("State(s) at Back (\"\")")) -> ("States Out"=w530:string)  [unwired: 13 in]
      }
      frame "Mercury: Query ITC: System" {
        n251 = Unbundle By Name(w573) -> ("Mercury ITC Ref"=w533:T50)
        n252 = call-poly <instrlib>:"Configuration (Read).vi"("error in"=w537, "Mercury Reference In"=w533) -> ("error out"=w569:errorcluster, "Devices"=→"ITC Devices":string[], "Mercury Reference Out"=w570:T46)  [unwired: 1 in, 6 out]
        n253 = call-poly <instrlib>:"Configuration (Read).vi"("error in"=w569, "Mercury Reference In"=w570) -> ("error out"=w562:errorcluster, "Automatic Dimming"=→"Automatic Dimming":string, "Mercury Reference Out"=w563:T46)  [unwired: 1 in, 6 out]
        n254 = call-poly <instrlib>:"Configuration (Read).vi"("error in"=w562, "Mercury Reference In"=w563) -> ("error out"=w565:errorcluster, "Dimming Time"=→"Dimming Time":string, "Mercury Reference Out"=w564:T46)  [unwired: 1 in, 6 out]
        n255 = call-poly <instrlib>:"Configuration (Read).vi"("error in"=w565, "Mercury Reference In"=w564) -> ("error out"=w571:errorcluster, "Display Brightness"=→"Display Brightness":string, "Mercury Reference Out"=w572:T46)  [unwired: 1 in, 6 out]
        n256 = call-poly <instrlib>:"Configuration (Read).vi"("error in"=w571, "Mercury Reference In"=w572) -> ("error out"=w556:errorcluster, "Date"=→"Date":string, "Mercury Reference Out"=w555:T46)  [unwired: 1 in, 6 out]
        n257 = call-poly <instrlib>:"Configuration (Read).vi"("error in"=w556, "Mercury Reference In"=w555) -> ("error out"=w558:errorcluster, "Time"=→"Time":string, "Mercury Reference Out"=w557:T46)  [unwired: 1 in, 6 out]
        n258 = call-poly <instrlib>:"Configuration (Read).vi"("error in"=w558, "Mercury Reference In"=w557) -> ("error out"=w536:errorcluster, "time stamp"=→"time stamp":timestamp, "Mercury Reference Out"=w534:T46)  [unwired: 1 in, 6 out]
        n259 = call-poly <instrlib>:"Configuration (Read).vi"("error in"=w536, "Mercury Reference In"=w534) -> ("error out"=w554:errorcluster, "Hardware Version"=→"Hardware Version":string, "Mercury Reference Out"=w553:T46)  [unwired: 1 in, 6 out]
        n260 = call-poly <instrlib>:"Configuration (Read).vi"("error in"=w554, "Mercury Reference In"=w553) -> ("error out"=w552:errorcluster, "Firmware Version"=→"Firmware Version":string, "Mercury Reference Out"=w551:T46)  [unwired: 1 in, 6 out]
        n261 = call-poly <instrlib>:"Configuration (Read).vi"("error in"=w552, "Mercury Reference In"=w551) -> ("error out"=w539:errorcluster, "Serial Number"=→"Serial Number":string, "Mercury Reference Out"=w538:T46)  [unwired: 1 in, 6 out]
        n262 = call-poly <instrlib>:"Configuration (Read).vi"("error in"=w539, "Mercury Reference In"=w538) -> ("error out"=w545:errorcluster, "Free Space"=→"Free Space":i32, "Mercury Reference Out"=w544:T46)  [unwired: 1 in, 6 out]
        n263 = call-poly <instrlib>:"Configuration (Read).vi"("error in"=w545, "Mercury Reference In"=w544) -> ("error out"=w541:errorcluster, "Mode"=→"String":T53, "Mercury Reference Out"=w542:T46)  [unwired: 1 in, 6 out]
        n264 = Get Date/Time In Seconds() -> (seconds since 1Jan1904=w550:timestamp)
        n265 = call-poly <instrlib>:"Configuration (Set).vi"("error in"=w541, "time stamp"=w550, "Mercury Reference In"=w542) -> ("error out"=w535:errorcluster, "Response"=→"Set Date Response":T48)  [unwired: 1 in, 6 out]
        n266 = call <vilib>:"Add State(s) to Queue__JKI_lib_State_Machine.vi"("State(s) in (\"\")"=w575) -> ("States Out"=w574:string)  [unwired: 14 in]
      }
      frame "Mercury: Query ITC: Temperature" {
        # "Temperature"
        n267 = Unbundle By Name(w620) -> ("Mercury ITC Ref"=w577:T50)
        n268 = local read "ITC Devices"() -> (w576:string[])
        n269 = Index Array(array=w576, index=3) -> (element=w578:string)
        n270 = call-poly <instrlib>:"Open.vi"("error in (no error)"=w583, "Device Identifier"=w578, "Mercury Reference In"=w577) -> ("error out"=w595:errorcluster, "Mercury Reference Out"=w596:T46)  [unwired: 7 out]
        n271 = call-poly <instrlib>:"Configuration (Read).vi"("error in"=w595, "Mercury Reference In"=w596) -> ("error out"=w587:errorcluster, "Serial Number"=→"Temp S/N":string, "Mercury Reference Out"=w586:T46)  [unwired: 1 in, 6 out]
        n272 = call-poly <instrlib>:"Configuration (Read).vi"("error in"=w587, "Mercury Reference In"=w586) -> ("error out"=w589:errorcluster, "Nickname"=→"T Nickname":string, "Mercury Reference Out"=w588:T46)  [unwired: 1 in, 6 out]
        n273 = call-poly <instrlib>:"Configuration (Read).vi"("error in"=w589, "Mercury Reference In"=w588) -> ("error out"=w592:errorcluster, "Unit"=→"Unit":T3, "Excitation Magnitude"=→"Excitation Magnitude":dbl, "Mercury Reference Out"=w591:T46)  [unwired: 1 in, 5 out]
        n274 = call-poly <instrlib>:"Configuration (Read).vi"("error in"=w592, "Mercury Reference In"=w591) -> ("error out"=w581:errorcluster, "Sensor Type"=→"Sensor Type":T6, "Mercury Reference Out"=w579:T46)  [unwired: 1 in, 6 out]
        n275 = call-poly <instrlib>:"Configuration (Read).vi"("error in"=w581, "Mercury Reference In"=w579) -> ("error out"=w598:errorcluster, "Excitation Type"=→"Excitation Type":T8, "Mercury Reference Out"=w599:T46)  [unwired: 1 in, 6 out]
        n276 = call-poly <instrlib>:"Configuration (Read).vi"("error in"=w598, "Mercury Reference In"=w599) -> ("error out"=w600:errorcluster, "Unit"=→"H Unit":T3, "Hot Limit"=→"Hot Limit":dbl, "Mercury Reference Out"=w601:T46)  [unwired: 1 in, 5 out]
        n277 = call-poly <instrlib>:"Configuration (Read).vi"("error in"=w600, "Mercury Reference In"=w601) -> ("error out"=w607:errorcluster, "Unit"=→"C Unit":T3, "Cold Limit"=→"Cold Limit":dbl, "Mercury Reference Out"=w606:T46)  [unwired: 1 in, 5 out]
        n278 = call-poly <instrlib>:"Signals (Read).vi"("error in"=w607, "Mercury Reference In"=w606) -> ("error out"=w611:errorcluster, "Unit"=→"V Unit":T3, "Voltage"=→"Voltage":dbl, "Mercury Reference Out"=w610:T46)  [unwired: 1 in, 5 out]
        n279 = call-poly <instrlib>:"Signals (Read).vi"("error in"=w611, "Mercury Reference In"=w610) -> ("error out"=w612:errorcluster, "Unit"=→"T Unit":T3, "Temperature"=→"Temperature":dbl, "Mercury Reference Out"=w615:T46)  [unwired: 1 in, 5 out]
        n280 = call-poly <instrlib>:"Configuration (Read).vi"("error in"=w612, "Mercury Reference In"=w615) -> ("error out"=w618:errorcluster, "Device Details"=→"Temperature Device Settings":T4, "Mercury Reference Out"=w617:T46)  [unwired: 1 in, 6 out]
        n281 = call-poly <instrlib>:"Configuration (Read).vi"("error in"=w618, "Mercury Reference In"=w617) -> ("error out"=w582:errorcluster, "Loop Details"=→"T Loop Details":T11)  [unwired: 1 in, 7 out]
        n282 = call <vilib>:"Add State(s) to Queue__JKI_lib_State_Machine.vi"("State(s) in (\"\")"=w621) -> ("States Out"=w622:string)  [unwired: 14 in]
      }
      frame "Mercury: Query ITC: Heater" {
        # "Heater"
        n283 = Unbundle By Name(w627) -> ("Mercury ITC Ref"=w626:T50)
        n284 = local read "ITC Devices"() -> (w628:string[])
        n285 = Index Array(array=w628, index=2) -> (element=w623:string)
        n286 = call-poly <instrlib>:"Open.vi"("error in (no error)"=w630, "Device Identifier"=w623, "Mercury Reference In"=w626) -> ("error out"=w633:errorcluster, "Mercury Reference Out"=w632:T46)  [unwired: 7 out]
        n287 = call-poly <instrlib>:"Configuration (Read).vi"("error in"=w633, "Mercury Reference In"=w632) -> ("error out"=w640:errorcluster, "Device Details"=→"Heater Device Settings":T13, "Mercury Reference Out"=w639:T46)  [unwired: 1 in, 6 out]
        n288 = call-poly <instrlib>:"Configuration (Read).vi"("error in"=w640, "Mercury Reference In"=w639) -> ("error out"=w642:errorcluster, "Nickname"=→"Htr Nickname":string, "Mercury Reference Out"=w641:T46)  [unwired: 1 in, 6 out]
        n289 = call-poly <instrlib>:"Configuration (Read).vi"("error in"=w642, "Mercury Reference In"=w641) -> ("error out"=w635:errorcluster, "Serial Number"=→"Htr S/N":string, "Mercury Reference Out"=w634:T46)  [unwired: 1 in, 6 out]
        n290 = call-poly <instrlib>:"Configuration (Read).vi"("error in"=w635, "Mercury Reference In"=w634) -> ("error out"=w631:errorcluster, "Unit"=→"Volt Unit":T3, "Voltage Limit"=→"Htr Voltage Limit":dbl, "Mercury Reference Out"=w625:T46)  [unwired: 1 in, 5 out]
        n291 = call-poly <instrlib>:"Configuration (Read).vi"("error in"=w631, "Mercury Reference In"=w625) -> ("error out"=w645:errorcluster, "Unit"=→"Res Unit":T3, "Nominal Resistance"=→"Htr Resistance":dbl, "Mercury Reference Out"=w646:T46)  [unwired: 1 in, 5 out]
        n292 = call-poly <instrlib>:"Configuration (Read).vi"("error in"=w645, "Mercury Reference In"=w646) -> ("error out"=w652:errorcluster, "Unit"=→"Power Unit":T3, "Maximum Power"=→"Maximum Power":dbl, "Mercury Reference Out"=w651:T46)  [unwired: 1 in, 5 out]
        n293 = call-poly <instrlib>:"Signals (Read).vi"("error in"=w652, "Mercury Reference In"=w651) -> ("error out"=w654:errorcluster, "Unit"=→"Htr V Unit":T3, "Voltage"=→"Htr Voltage":dbl, "Mercury Reference Out"=w653:T46)  [unwired: 1 in, 5 out]
        n294 = call-poly <instrlib>:"Signals (Read).vi"("error in"=w654, "Mercury Reference In"=w653) -> ("error out"=w656:errorcluster, "Unit"=→"Htr P Unit":T3, "Power"=→"Htr Power":dbl, "Mercury Reference Out"=w655:T46)  [unwired: 1 in, 5 out]
        n295 = call-poly <instrlib>:"Signals (Read).vi"("error in"=w656, "Mercury Reference In"=w655) -> ("error out"=w624:errorcluster, "Unit"=→"Htr C Unit":T3, "Current"=→"Htr Current":dbl)  [unwired: 1 in, 6 out]
        n296 = call <vilib>:"Add State(s) to Queue__JKI_lib_State_Machine.vi"("State(s) in (\"\")"=w663) -> ("States Out"=w664:string)  [unwired: 14 in]
      }
      frame "Mercury: Query ITC: Aux" {
        # "Auxiliary"
        n297 = Unbundle By Name(w670) -> ("Mercury ITC Ref"=w665:T50)
        n298 = local read "ITC Devices"() -> (w668:string[])
        n299 = Index Array(array=w668, index=0) -> (element=w666:string)
        n300 = call-poly <instrlib>:"Open.vi"("error in (no error)"=w672, "Device Identifier"=w666, "Mercury Reference In"=w665) -> ("error out"=w692:errorcluster, "Mercury Reference Out"=w693:T46)  [unwired: 7 out]
        n301 = call-poly <instrlib>:"Configuration (Read).vi"("error in"=w692, "Mercury Reference In"=w693) -> ("error out"=w696:errorcluster, "Auxiliary Device Details"=→"Auxiliary Device Details":T21, "Mercury Reference Out"=w695:T46)  [unwired: 1 in, 6 out]
        n302 = call-poly <instrlib>:"Configuration (Read).vi"("error in"=w696, "Mercury Reference In"=w695) -> ("error out"=w699:errorcluster, "Serial Number"=→"Aux S/N":string, "Mercury Reference Out"=w698:T46)  [unwired: 1 in, 6 out]
        n303 = call-poly <instrlib>:"Configuration (Read).vi"("error in"=w699, "Mercury Reference In"=w698) -> ("error out"=w701:errorcluster, "Unit"=→"Unit 2":T3, "Min Flow"=→"Min Flow":dbl, "Mercury Reference Out"=w700:T46)  [unwired: 1 in, 5 out]
        n304 = call-poly <instrlib>:"Configuration (Read).vi"("error in"=w701, "Mercury Reference In"=w700) -> ("error out"=w703:errorcluster, "Unit"=→"Unit 3":T3, "Scaling Factor"=→"Scaling Factor":dbl, "Mercury Reference Out"=w702:T46)  [unwired: 1 in, 5 out]
        n305 = call-poly <instrlib>:"Configuration (Read).vi"("error in"=w703, "Mercury Reference In"=w702) -> ("error out"=w671:errorcluster, "Unit"=→"Unit 4":T3, "Temp Err"=→"Temp Err":dbl, "Mercury Reference Out"=w667:T46)  [unwired: 1 in, 5 out]
        n306 = call-poly <instrlib>:"Configuration (Read).vi"("error in"=w671, "Mercury Reference In"=w667) -> ("error out"=w675:errorcluster, "Unit"=→"Unit 5":T3, "Temp V Err"=→"Temp V Err":dbl, "Mercury Reference Out"=w674:T46)  [unwired: 1 in, 5 out]
        n307 = call-poly <instrlib>:"Configuration (Read).vi"("error in"=w675, "Mercury Reference In"=w674) -> ("error out"=w677:errorcluster, "Unit"=→"Unit 6":T3, "Gear"=→"Gear":u32, "Mercury Reference Out"=w676:T46)  [unwired: 1 in, 5 out]
        n308 = call-poly <instrlib>:"Configuration (Read).vi"("error in"=w677, "Mercury Reference In"=w676) -> ("error out"=w685:errorcluster, "Unit"=→"Unit 7":T3, "Speed"=→"Speed":u32, "Mercury Reference Out"=w684:T46)  [unwired: 1 in, 5 out]
        n309 = call-poly <instrlib>:"Signals (Read).vi"("error in"=w685, "Mercury Reference In"=w684) -> ("error out"=w687:errorcluster, "Unit"=→"Unit":T3, "Position"=→"Position":u32, "Mercury Reference Out"=w686:T46)  [unwired: 1 in, 5 out]
        n310 = call-poly <instrlib>:"Signals (Read).vi"("error in"=w687, "Mercury Reference In"=w686) -> ("error out"=w673:errorcluster, "Unit"=→"Unit":T3, "% Open"=→"% Open":dbl)  [unwired: 1 in, 6 out]
        n311 = call <vilib>:"Add State(s) to Queue__JKI_lib_State_Machine.vi"("State(s) in (\"\")"=w710) -> ("States Out"=w711:string)  [unwired: 14 in]
      }
      frame "Mercury: Query ITC: Pressure" {
        # "Pressure"
        n312 = Unbundle By Name(w717) -> ("Mercury ITC Ref"=w714:T50)
        n313 = local read "ITC Devices"() -> (w716:string[])
        n314 = Index Array(array=w716, index=1) -> (element=w713:string)
        n315 = call-poly <instrlib>:"Open.vi"("error in (no error)"=w712, "Device Identifier"=w713, "Mercury Reference In"=w714) -> ("error out"=w720:errorcluster, "Mercury Reference Out"=w721:T46)  [unwired: 7 out]
        n316 = call-poly <instrlib>:"Configuration (Read).vi"("error in"=w720, "Mercury Reference In"=w721) -> ("error out"=w722:errorcluster, "Device Details"=→"Pressure Device":T15, "Mercury Reference Out"=w723:T46)  [unwired: 1 in, 6 out]
        n317 = call-poly <instrlib>:"Configuration (Read).vi"("error in"=w722, "Mercury Reference In"=w723) -> ("error out"=w727:errorcluster, "Nickname"=→"Nickname":string, "Mercury Reference Out"=w728:T46)  [unwired: 1 in, 6 out]
        n318 = call-poly <instrlib>:"Signals (Read).vi"("error in"=w727, "Mercury Reference In"=w728) -> ("error out"=w725:errorcluster, "Current"=→"Current":dbl, "Mercury Reference Out"=w726:T46)  [unwired: 1 in, 6 out]
        n319 = call-poly <instrlib>:"Signals (Read).vi"("error in"=w725, "Mercury Reference In"=w726) -> ("error out"=w718:errorcluster, "Voltage"=→"Voltage":dbl)  [unwired: 1 in, 7 out]
        n320 = call <vilib>:"Add State(s) to Queue__JKI_lib_State_Machine.vi"("State(s) in (\"\")"=w731) -> ("States Out"=w732:string)  [unwired: 14 in]
      }
      frame "Mercury: Query IPS: System" {
        # "Your code here.\n(You can make a copy of, or modify, this frame)"
        n321 = Unbundle By Name(w774) -> ("Mercury IPS Ref"=w735:T46)
        n322 = call-poly <instrlib>:"Configuration (Read).vi"("error in"=w740, "Mercury Reference In"=w735) -> ("error out"=w760:errorcluster, "Devices"=→"IPS Devices":string[], "Mercury Reference Out"=w759:T46)  [unwired: 1 in, 6 out]
        n323 = call-poly <instrlib>:"Configuration (Read).vi"("error in"=w760, "Mercury Reference In"=w759) -> ("error out"=w764:errorcluster, "Automatic Dimming"=→"Automatic Dimming 2":string, "Mercury Reference Out"=w763:T46)  [unwired: 1 in, 6 out]
        n324 = call-poly <instrlib>:"Configuration (Read).vi"("error in"=w764, "Mercury Reference In"=w763) -> ("error out"=w761:errorcluster, "Dimming Time"=→"Dimming Time 2":string, "Mercury Reference Out"=w762:T46)  [unwired: 1 in, 6 out]
        n325 = call-poly <instrlib>:"Configuration (Read).vi"("error in"=w761, "Mercury Reference In"=w762) -> ("error out"=w758:errorcluster, "Display Brightness"=→"Display Brightness 2":string, "Mercury Reference Out"=w757:T46)  [unwired: 1 in, 6 out]
        n326 = call-poly <instrlib>:"Configuration (Read).vi"("error in"=w758, "Mercury Reference In"=w757) -> ("error out"=w767:errorcluster, "Date"=→"Date 2":string, "Mercury Reference Out"=w768:T46)  [unwired: 1 in, 6 out]
        n327 = call-poly <instrlib>:"Configuration (Read).vi"("error in"=w767, "Mercury Reference In"=w768) -> ("error out"=w765:errorcluster, "Time"=→"Time 2":string, "Mercury Reference Out"=w766:T46)  [unwired: 1 in, 6 out]
        n328 = call-poly <instrlib>:"Configuration (Read).vi"("error in"=w765, "Mercury Reference In"=w766) -> ("error out"=w739:errorcluster, "time stamp"=→"time stamp 2":timestamp, "Mercury Reference Out"=w736:T46)  [unwired: 1 in, 6 out]
        n329 = call-poly <instrlib>:"Configuration (Read).vi"("error in"=w739, "Mercury Reference In"=w736) -> ("error out"=w741:errorcluster, "Hardware Version"=→"Hardware Version 2":string, "Mercury Reference Out"=w742:T46)  [unwired: 1 in, 6 out]
        n330 = call-poly <instrlib>:"Configuration (Read).vi"("error in"=w741, "Mercury Reference In"=w742) -> ("error out"=w743:errorcluster, "Firmware Version"=→"Firmware Version 2":string, "Mercury Reference Out"=w744:T46)  [unwired: 1 in, 6 out]
        n331 = call-poly <instrlib>:"Configuration (Read).vi"("error in"=w743, "Mercury Reference In"=w744) -> ("error out"=w749:errorcluster, "Serial Number"=→"Serial Number 2":string, "Mercury Reference Out"=w750:T46)  [unwired: 1 in, 6 out]
        n332 = call-poly <instrlib>:"Configuration (Read).vi"("error in"=w749, "Mercury Reference In"=w750) -> ("error out"=w745:errorcluster, "Free Space"=→"Free Space 2":i32, "Mercury Reference Out"=w746:T46)  [unwired: 1 in, 6 out]
        n333 = call-poly <instrlib>:"Configuration (Read).vi"("error in"=w745, "Mercury Reference In"=w746) -> ("error out"=w748:errorcluster, "Mode"=→"String 2":T53, "Mercury Reference Out"=w747:T46)  [unwired: 1 in, 6 out]
        n334 = Get Date/Time In Seconds() -> (seconds since 1Jan1904=w756:timestamp)
        n335 = call-poly <instrlib>:"Configuration (Set).vi"("error in"=w748, "time stamp"=w756, "Mercury Reference In"=w747) -> ("error out"=w738:errorcluster, "Response"=→"Set Date Response 2":T48)  [unwired: 1 in, 6 out]
        n336 = call <vilib>:"Add State(s) to Queue__JKI_lib_State_Machine.vi"("State(s) in (\"\")"=w776) -> ("States Out"=w775:string)  [unwired: 14 in]
      }
      frame "Mercury: Query IPS: LVL" {
        # "Level"
        n337 = Unbundle By Name(w816) -> ("Mercury IPS Ref"=w779:T46)
        n338 = local read "IPS Devices"() -> (w815:string[])
        n339 = Index Array(array=w815, index=0) -> (element=w778:string)
        n340 = call-poly <instrlib>:"Open.vi"("error in (no error)"=w785, "Device Identifier"=w778, "Mercury Reference In"=w779) -> ("error out"=w801:errorcluster, "Mercury Reference Out"=w800:T46)  [unwired: 7 out]
        n341 = call-poly <instrlib>:"Configuration (Read).vi"("error in"=w801, "Mercury Reference In"=w800) -> ("error out"=w806:errorcluster, "LVL Device Settings"=→"LVL Device DetailSettings":T23, "Mercury Reference Out"=w803:T46)  [unwired: 1 in, 6 out]
        n342 = call-poly <instrlib>:"Configuration (Read).vi"("error in"=w806, "Mercury Reference In"=w803) -> ("error out"=w807:errorcluster, "Serial Number"=→"LVL S/N":string, "Mercury Reference Out"=w805:T46)  [unwired: 1 in, 6 out]
        n343 = call-poly <instrlib>:"Configuration (Read).vi"("error in"=w807, "Mercury Reference In"=w805) -> ("error out"=w810:errorcluster, "Resistance Configuration"=→"He Res Config":T28, "Mercury Reference Out"=w809:T46)  [unwired: 1 in, 6 out]
        n344 = call-poly <instrlib>:"Configuration (Read).vi"("error in"=w810, "Mercury Reference In"=w809) -> ("error out"=w812:errorcluster, "Magnitude"=→"LVL P Magnitude":dbl, "Mercury Reference Out"=w811:T46)  [unwired: 1 in, 6 out]
        n345 = call-poly <instrlib>:"Configuration (Read).vi"("error in"=w812, "Mercury Reference In"=w811) -> ("error out"=w784:errorcluster, "Duration"=→"LVL P Duration":dbl, "Mercury Reference Out"=w782:T46)  [unwired: 1 in, 6 out]
        n346 = call-poly <instrlib>:"Configuration (Read).vi"("error in"=w784, "Mercury Reference In"=w782) -> ("error out"=w788:errorcluster, "Freq 100%"=→"N Freq 100%":dbl, "Mercury Reference Out"=w787:T46)  [unwired: 1 in, 6 out]
        n347 = call-poly <instrlib>:"Configuration (Read).vi"("error in"=w788, "Mercury Reference In"=w787) -> ("error out"=w791:errorcluster, "Pulse Period"=→"N Pulse Period":dbl, "Mercury Reference Out"=w790:T46)  [unwired: 1 in, 6 out]
        n348 = call-poly <instrlib>:"Signals (Read).vi"("error in"=w791, "Mercury Reference In"=w790) -> ("error out"=w793:errorcluster, "Resistance"=→"He Resistance":dbl, "Mercury Reference Out"=w792:T46)  [unwired: 1 in, 6 out]
        n349 = call-poly <instrlib>:"Signals (Read).vi"("error in"=w793, "Mercury Reference In"=w792) -> ("error out"=w795:errorcluster, "Level"=→"He Level" →"He LEVEL":dbl, "Mercury Reference Out"=w794:T46)  [unwired: 1 in, 6 out]
        n350 = call-poly <instrlib>:"Signals (Read).vi"("error in"=w795, "Mercury Reference In"=w794) -> ("error out"=w797:errorcluster, "Counter"=→"N Counter":u32, "Mercury Reference Out"=w796:T46)  [unwired: 1 in, 6 out]
        n351 = call-poly <instrlib>:"Signals (Read).vi"("error in"=w797, "Mercury Reference In"=w796) -> ("error out"=w783:errorcluster, "Level"=→"N Level" →"N2 LEVEL":dbl)  [unwired: 1 in, 7 out]
        n352 = call <vilib>:"Add State(s) to Queue__JKI_lib_State_Machine.vi"("State(s) in (\"\")"=w817) -> ("States Out"=w818:string)  [unwired: 14 in]
      }
      frame "Mercury: Query IPS: Temperature" {
        n353 = Unbundle By Name(w863) -> ("Mercury IPS Ref"=w820:T46)
        n354 = local read "IPS Devices"() -> (w862:string[])
        n355 = Index Array(array=w862, index=4) -> (element=w821:string)
        n356 = call-poly <instrlib>:"Open.vi"("error in (no error)"=w819, "Device Identifier"=w821, "Mercury Reference In"=w820) -> ("error out"=w850:errorcluster, "Mercury Reference Out"=w845:T46)  [unwired: 7 out]
        n357 = call-poly <instrlib>:"Configuration (Read).vi"("error in"=w850, "Mercury Reference In"=w845) -> ("error out"=w851:errorcluster, "Serial Number"=→"Temp S/N 2":string, "Mercury Reference Out"=w846:T46)  [unwired: 1 in, 6 out]
        n358 = call-poly <instrlib>:"Configuration (Read).vi"("error in"=w851, "Mercury Reference In"=w846) -> ("error out"=w852:errorcluster, "Nickname"=→"T Nickname 2":string, "Mercury Reference Out"=w847:T46)  [unwired: 1 in, 6 out]
        n359 = call-poly <instrlib>:"Configuration (Read).vi"("error in"=w852, "Mercury Reference In"=w847) -> ("error out"=w853:errorcluster, "Unit"=→"Unit 12":T3, "Excitation Magnitude"=→"Excitation Magnitude 2":dbl, "Mercury Reference Out"=w848:T46)  [unwired: 1 in, 5 out]
        n360 = call-poly <instrlib>:"Configuration (Read).vi"("error in"=w853, "Mercury Reference In"=w848) -> ("error out"=w854:errorcluster, "Sensor Type"=→"Sensor Type 2":T6, "Mercury Reference Out"=w849:T46)  [unwired: 1 in, 6 out]
        n361 = call-poly <instrlib>:"Configuration (Read).vi"("error in"=w854, "Mercury Reference In"=w849) -> ("error out"=w824:errorcluster, "Excitation Type"=→"Excitation Type 2":T8, "Mercury Reference Out"=w823:T46)  [unwired: 1 in, 6 out]
        n362 = call-poly <instrlib>:"Configuration (Read).vi"("error in"=w824, "Mercury Reference In"=w823) -> ("error out"=w830:errorcluster, "Unit"=→"H Unit 2":T3, "Hot Limit"=→"Hot Limit 2":dbl, "Mercury Reference Out"=w825:T46)  [unwired: 1 in, 5 out]
        n363 = call-poly <instrlib>:"Configuration (Read).vi"("error in"=w830, "Mercury Reference In"=w825) -> ("error out"=w831:errorcluster, "Unit"=→"C Unit 2":T3, "Cold Limit"=→"Cold Limit 2":dbl, "Mercury Reference Out"=w826:T46)  [unwired: 1 in, 5 out]
        n364 = call-poly <instrlib>:"Signals (Read).vi"("error in"=w831, "Mercury Reference In"=w826) -> ("error out"=w832:errorcluster, "Unit"=→"V Unit 2":T3, "Voltage"=→"Voltage 2":dbl, "Mercury Reference Out"=w827:T46)  [unwired: 1 in, 5 out]
        n365 = call-poly <instrlib>:"Signals (Read).vi"("error in"=w832, "Mercury Reference In"=w827) -> ("error out"=w833:errorcluster, "Unit"=→"T Unit 2":T3, "Temperature"=→"Temperature 2":dbl, "Mercury Reference Out"=w828:T46)  [unwired: 1 in, 5 out]
        n366 = call-poly <instrlib>:"Configuration (Read).vi"("error in"=w833, "Mercury Reference In"=w828) -> ("error out"=w834:errorcluster, "Device Details"=→"Temperature Device Settings 2":T4, "Mercury Reference Out"=w829:T46)  [unwired: 1 in, 6 out]
        n367 = call-poly <instrlib>:"Configuration (Read).vi"("error in"=w834, "Mercury Reference In"=w829) -> ("error out"=w822:errorcluster, "Loop Details"=→"T Loop Details 2":T11)  [unwired: 1 in, 7 out]
        n368 = call <vilib>:"Add State(s) to Queue__JKI_lib_State_Machine.vi"("State(s) in (\"\")"=w864) -> ("States Out"=w865:string)  [unwired: 14 in]
      }
      frame "Mercury: Query IPS: Magnet" {
        n369 = Unbundle By Name(w904) -> ("Mercury IPS Ref"=w870:T46)
        n370 = call-poly <instrlib>:"Open.vi"("error in (no error)"=w866, "Device Identifier"="Device Identifier", "Mercury Reference In"=w870) -> ("error out"=w889:errorcluster, "Mercury Reference Out"=w888:T46)  [unwired: 7 out]
        n371 = call-poly <instrlib>:"Configuration (Read).vi"("error in"=w889, "Mercury Reference In"=w888) -> ("error out"=w892:errorcluster, "Magnet Device Details"=→"Magnet Device Details":T31, "Mercury Reference Out"=w891:T46)  [unwired: 1 in, 6 out]
        n372 = call-poly <instrlib>:"Configuration (Read).vi"("error in"=w892, "Mercury Reference In"=w891) -> ("error out"=w895:errorcluster, "Serial Number"=→"Mag S/N":string, "Mercury Reference Out"=w894:T46)  [unwired: 1 in, 6 out]
        n373 = call-poly <instrlib>:"Configuration (Read).vi"("error in"=w895, "Mercury Reference In"=w894) -> ("error out"=w898:errorcluster, "Bipolar Output"=→"Bipolar Output":string, "Mercury Reference Out"=w897:T46)  [unwired: 1 in, 6 out]
        n374 = call-poly <instrlib>:"Configuration (Read).vi"("error in"=w898, "Mercury Reference In"=w897) -> ("error out"=w901:errorcluster, "Out Config"=→"Out Config":T54, "Mercury Reference Out"=w900:T46)  [unwired: 1 in, 6 out]
        n375 = call-poly <instrlib>:"Configuration (Read).vi"("error in"=w901, "Mercury Reference In"=w900) -> ("error out"=w872:errorcluster, "Unit"=→"Unit 8":T3, "Current Limit"=→"Current Limit":dbl, "Mercury Reference Out"=w869:T46)  [unwired: 1 in, 5 out]
        n376 = call-poly <instrlib>:"Configuration (Read).vi"("error in"=w872, "Mercury Reference In"=w869) -> ("error out"=w875:errorcluster, "Unit"=→"Unit 9":T3, "AtoB"=→"AtoB":dbl, "Mercury Reference Out"=w874:T46)  [unwired: 1 in, 5 out]
        n377 = call-poly <instrlib>:"Configuration (Read).vi"("error in"=w875, "Mercury Reference In"=w874) -> ("error out"=w878:errorcluster, "Switch Present"=→"Switch Present":string, "Mercury Reference Out"=w877:T46)  [unwired: 1 in, 6 out]
        n378 = call-poly <instrlib>:"Configuration (Read).vi"("error in"=w878, "Mercury Reference In"=w877) -> ("error out"=w883:errorcluster, "Unit"=→"Unit 10":T3, "SW VLIM"=→"SW VLIM":dbl, "Mercury Reference Out"=w882:T46)  [unwired: 1 in, 5 out]
        n379 = call-poly <instrlib>:"Signals (Read).vi"("error in"=w883, "Mercury Reference In"=w882) -> ("error out"=w885:errorcluster, "Unit"=→"Unit 11":T3, "Current Rate"=→"Current Rate":dbl, "Mercury Reference Out"=w884:T46)  [unwired: 1 in, 5 out]
        n380 = call-poly <instrlib>:"Signals (Read).vi"("error in"=w885, "Mercury Reference In"=w884) -> ("error out"=w871:errorcluster, "PSU Act Stat"=→"PSU Act Stat":T36)  [unwired: 1 in, 7 out]
        n381 = call <vilib>:"Add State(s) to Queue__JKI_lib_State_Machine.vi"("State(s) in (\"\")"=w905) -> ("States Out"=w906:string)  [unwired: 14 in]
      }
      frame "Mercury: IPS: Idle - 1" {
        n382 = Unbundle By Name(w947) -> ("Mercury IPS Ref"=w915:T46)
        n383 = local read "Device Identifier"() -> (w928:T33)
        n384 = call-poly <instrlib>:"Configuration (Read).vi"("error in"=w946, "Mercury Reference In"=w915) -> ("error out"=w935:errorcluster, "Time"=w939:string, "Mercury Reference Out"=w936:T46)  [unwired: 1 in, 6 out]
        n385 = local write "Time 2"(w939) -> ()
        n386 = call-poly <instrlib>:"Open.vi"("error in (no error)"=w935, "Device Identifier"=w928, "Mercury Reference In"=w936) -> ("error out"=w934:errorcluster, "Mercury Reference Out"=w933:T46)  [unwired: 7 out]
        n387 = call-poly <instrlib>:"Signals (Read).vi"("error in"=w934, "Mercury Reference In"=w933) -> ("error out"=w945:errorcluster, "Switch Heater Status"=w937:string, "Mercury Reference Out"=w942:T46)  [unwired: 1 in, 6 out]
        n388 = Equal?(x=w937, y="ON") -> (x = y?=w912:bool)
        "SWITCH HEATER" <- w912
        n389 = call-poly <instrlib>:"Signals (Read).vi"("error in"=w945, "Mercury Reference In"=w942) -> ("error out"=w944:errorcluster, "Current"=→"Current (A)" →"Current (A)":dbl, "Mercury Reference Out"=w941:T46)  [unwired: 1 in, 6 out]
        n390 = call-poly <instrlib>:"Signals (Read).vi"("error in"=w944, "Mercury Reference In"=w941) -> ("error out"=w927:errorcluster, "Voltage"=→"Voltage (V)" →"Voltage (V)":dbl, "Mercury Reference Out"=w926:T46)  [unwired: 1 in, 6 out]
        n391 = call-poly <instrlib>:"Signals (Read).vi"("error in"=w927, "Mercury Reference In"=w926) -> ("error out"=w929:errorcluster, "Field"=→"Power Supply Field (T)":dbl, "Mercury Reference Out"=w932:T46)  [unwired: 1 in, 6 out]
        n392 = call-poly <instrlib>:"Signals (Read).vi"("error in"=w929, "Mercury Reference In"=w932) -> ("error out"=w930:errorcluster, "Target Field Rate"=→"Target Field Rate (T/min)":dbl, "Mercury Reference Out"=w931:T46)  [unwired: 1 in, 6 out]
        n393 = call-poly <instrlib>:"Signals (Read).vi"("error in"=w930, "Mercury Reference In"=w931) -> ("error out"=w925:errorcluster, "Target Field"=→"Target Field (T)":dbl, "Mercury Reference Out"=w924:T46)  [unwired: 1 in, 6 out]
        n394 = call-poly <instrlib>:"Signals (Read).vi"("error in"=w925, "Mercury Reference In"=w924) -> ("error out"=w943:errorcluster, "Persistant Field"=→"Magnet Field (T)" →"Magnet Field (T)":dbl, "Mercury Reference Out"=w940:T46)  [unwired: 1 in, 6 out]
        n395 = call-poly <instrlib>:"Signals (Read).vi"("error in"=w943, "Mercury Reference In"=w940) -> ("error out"=w909:errorcluster, "PSU Act Stat"=w916:T36)  [unwired: 1 in, 7 out]
        n396 = call "FGV_PSP - Mercury Status.vi"("error in"=w909, "Function"=enum16{"write", "read"}."read") -> ("error out"=w911:errorcluster, "status"=w908:T55)  [unwired: 4 in]
        n397 = local write "PSU Act Stat"(w916) -> ()
        n398 = Bundle By Name(cluster=w908, "Switch"=w912) -> (w907:T55)
        n399 = case shown="\"CLMP\"" w916 {
          selector: w916 -> [w950 _ _ _ _]
          tunnel: [w950 "Holding" "Ramping to Setpoint" "Ramping to Zero" "Clamped"] -> w923
          frame Default {
          }
          frame "HOLD" {
          }
          frame "RTOS" {
          }
          frame "RTOZ" {
          }
          frame "CLMP" {
          }
        }
        "Magnet Status" <- w923
        n400 = call "FGV_PSP - Mercury Status.vi"("error in"=w911, "Function"=enum16{"write", "read"}."write", "status"=w907) -> ("error out"=w910:errorcluster)  [unwired: 3 in, 1 out]
        n401 = call <vilib>:"Add State(s) to Queue__JKI_lib_State_Machine.vi"("State(s) in (\"\")"=w948) -> ("States Out"=w949:string)  [unwired: 14 in]
      }
      frame "Mercury: IPS: Idle - 2" {
        n402 = Unbundle By Name(w1004) -> ("Mercury IPS Ref"=w970:T46)
        n403 = local read "IPS Devices"() -> (w998:string[])
        n404 = Index Array(array=w998, index=0) -> (element=w997:string)
        n405 = call-poly <instrlib>:"Open.vi"("error in (no error)"=w983, "Device Identifier"=w997, "Mercury Reference In"=w970) -> ("error out"=w1000:errorcluster, "Mercury Reference Out"=w1001:T46)  [unwired: 7 out]
        n406 = call-poly <instrlib>:"Signals (Read).vi"("error in"=w1000, "Mercury Reference In"=w1001) -> ("error out"=w1002:errorcluster, "Level"=w972:dbl, "Mercury Reference Out"=w1003:T46)  [unwired: 1 in, 6 out]
        "He LVL Chart" <- w972
        n407 = Greater?(x=w972, y=20.0) -> (0:w980:bool)
        n408 = Greater?(x=w972, y=50.0) -> (0:w981:bool)
        n409 = call-poly <instrlib>:"Signals (Read).vi"("error in"=w1002, "Mercury Reference In"=w1003) -> ("error out"=w987:errorcluster, "Level"=w971:dbl)  [unwired: 1 in, 7 out]
        "N2 LVL Chart" <- w971
        n410 = case shown="False" w980 {
          tunnel: [w1012 u32 6618880] -> w968
          tunnel: w981 -> [w1013 _]
          frame False {
            n411 = case shown="True" w1013 {
              tunnel: [u32 16711680 u32 16776704] -> w1012
              frame False {
              }
              frame True {
              }
            }
          }
          frame True {
          }
        }
        n412 = local write "He LEVEL"(w972) -> ()
        n413 = local read "IPS Devices"() -> (w992:string[])
        n414 = property on="He LVL Chart" class="Slide (strict)"("Fill Color"=w968) -> ()  [unwired: 2 in, 2 out]
        n415 = property on="He LEVEL" class="DigNum (strict)"("NumText.TextColor"=w968) -> ()  [unwired: 2 in, 2 out]
        n416 = local write "N2 LEVEL"(w971) -> ()
        n417 = Index Array(array=w992, index=4) -> (element=w990:string)
        n418 = local read "Target Field Rate (T/min)"() -> (w959:dbl)
        n419 = local read "Power Supply Field (T)"() -> (w957:dbl)
        n420 = call-poly <instrlib>:"Open.vi"("error in (no error)"=w987, "Device Identifier"=w990, "Mercury Reference In"=w970) -> ("error out"=w989:errorcluster, "Mercury Reference Out"=w988:T46)  [unwired: 7 out]
        n421 = Greater?(x=w971, y=20.0) -> (0:w974:bool)
        n422 = Greater?(x=w971, y=50.0) -> (0:w973:bool)
        n423 = local read "Magnet Field (T)"() -> (w956:dbl)
        n424 = local read "Target Field (T)"() -> (w958:dbl)
        n425 = local read "Current (A)"() -> (w961:dbl)
        n426 = local read "Voltage (V)"() -> (w960:dbl)
        n427 = case shown="False" w974 {
          tunnel: [w1007 u32 6618880] -> w969
          tunnel: w973 -> [w1008 _]
          frame False {
            n428 = case shown="True" w1008 {
              tunnel: [u32 16711680 u32 16776704] -> w1007
              frame False {
              }
              frame True {
              }
            }
          }
          frame True {
          }
        }
        n429 = call-poly <instrlib>:"Signals (Read).vi"("error in"=w989, "Mercury Reference In"=w988) -> ("error out"=w965:errorcluster, "Temperature"=w984:dbl)  [unwired: 1 in, 7 out]
        "Magnet Temperature" <- w984
        n430 = property on="N2 LVL Chart" class="Slide (strict)"("Fill Color"=w969) -> ()  [unwired: 2 in, 2 out]
        n431 = property on="N2 LEVEL" class="DigNum (strict)"("NumText.TextColor"=w969) -> ()  [unwired: 2 in, 2 out]
        n432 = local read "PSU Act Stat"() -> (w979:string)
        n433 = call "FGV_PSP - Mercury Status.vi"("error in"=w965, "Function"=enum16{"write", "read"}."read") -> ("error out"=w964:errorcluster, "status"=w962:T55)  [unwired: 4 in]
        n434 = Bundle By Name(cluster=w962, "Magnet Field"=w956, "PS Field"=w957, "Target Field"=w958, "Target Field Rate"=w959, "Voltage"=w960, "Current"=w961) -> (w963:T55)
        n435 = call "FGV_PSP - Mercury Status.vi"("error in"=w964, "Function"=enum16{"write", "read"}."write", "status"=w963) -> ("error out"=w985:errorcluster)  [unwired: 3 in, 1 out]
        n436 = Bundle(cluster=T43 {"Magnet Field"=0.0, "PS Field"=0.0, "Target Field"=0.0, "Target Field Rate"=0.0, "Voltage"=0.0, "Current"=0.0}, "Magnet Field"=w956, "PS Field"=w957, "Target Field"=w958, "Target Field Rate"=w959, "Voltage"=w960, "Current"=w961) -> (w967:T43)
        n437 = call "FGV_PSP - Mercury Action Status.vi"("error in"=w985, "Function"=enum16{"write", "read"}."write", "Mercury Status"=w979) -> ("error out"=w982:errorcluster)  [unwired: 3 in, 1 out]
        n438 = Cluster To Array(cluster=w967) -> (array=w994:dbl[])
        n439 = Build Array (concatenate)(w994, w971, w972, w984) -> (w993:dbl[])
        n440 = Build Array(w979) -> (w986:string[])
        n441 = call "1820_IPS_to_DSC.vi"("str"=w986, "dbl"=w993) -> ()  [unwired: 2 in]
        n442 = call <vilib>:"Add State(s) to Queue__JKI_lib_State_Machine.vi"("State(s) in (\"\")"=w1005) -> ("States Out"=w1006:string)  [unwired: 14 in]
      }
      frame "Mercury: ITC: Idle" {
        n443 = Unbundle By Name(w1043) -> ("Mercury ITC Ref"=w1023:T50)
        n444 = local read "ITC Devices"() -> (w1039:string[])
        n445 = Index Array(array=w1039, index=3) -> (element=w1038:string)
        n446 = call-poly <instrlib>:"Open.vi"("error in (no error)"=w1018, "Device Identifier"=w1038, "Mercury Reference In"=w1023) -> ("error out"=w1037:errorcluster, "Mercury Reference Out"=w1030:T46)  [unwired: 7 out]
        n447 = call-poly <instrlib>:"Signals (Read).vi"("error in"=w1037, "Mercury Reference In"=w1030) -> ("error out"=w1036:errorcluster, "Temperature"=w1021:dbl)  [unwired: 1 in, 7 out]
        "LPF Temperature" <- w1021
        n448 = local read "ITC Devices"() -> (w1042:string[])
        n449 = Index Array(array=w1042, index=1) -> (element=w1040:string)
        n450 = call-poly <instrlib>:"Open.vi"("error in (no error)"=w1036, "Device Identifier"=w1040, "Mercury Reference In"=w1023) -> ("error out"=w1035:errorcluster, "Mercury Reference Out"=w1034:T46)  [unwired: 7 out]
        n451 = call-poly <instrlib>:"Configuration (Read).vi"("error in"=w1035, "Mercury Reference In"=w1034) -> ("error out"=w1029:errorcluster, "Device Details"=w1033:T15)  [unwired: 1 in, 7 out]
        n452 = local read "ITC Devices"() -> (w1027:string[])
        n453 = Unbundle By Name(w1033) -> ("Pressure Signals.Pressure"=w1032:string)
        n454 = Index Array(array=w1027, index=0) -> (element=w1026:string)
        n455 = call-poly <instrlib>:"Open.vi"("error in (no error)"=w1029, "Device Identifier"=w1026, "Mercury Reference In"=w1023) -> ("error out"=w1025:errorcluster, "Mercury Reference Out"=w1024:T46)  [unwired: 7 out]
        n456 = Fract/Exp String To Number(string=w1032) -> (number=w1020:dbl)  [unwired: 3 in, 1 out]
        "LPF Pressure" <- w1020
        n457 = call-poly <instrlib>:"Signals (Read).vi"("error in"=w1025, "Mercury Reference In"=w1024) -> ("error out"=w1017:errorcluster, "% Open"=w1019:dbl)  [unwired: 1 in, 7 out]
        "LPF Needle Valve (%)" <- w1019
        n458 = Build Array(w1021, w1020, w1019) -> (w1022:dbl[])
        n459 = call "1820_ITC_to_DSC.vi"("dbl"=w1022) -> ()  [unwired: 3 in]
        n460 = call <vilib>:"Add State(s) to Queue__JKI_lib_State_Machine.vi"("State(s) in (\"\")"=w1044) -> ("States Out"=w1045:string)  [unwired: 14 in]
      }
      frame "Mercury: Empty" {
        n461 = Unbundle By Name(w1047) -> ()  [unwired: 1 out]
        n462 = call <vilib>:"Add State(s) to Queue__JKI_lib_State_Machine.vi"("State(s) in (\"\")"=w1048) -> ("States Out"=w1049:string)  [unwired: 14 in]
      }
      frame "Mercury: IPS: Idle - 3" {
        n463 = call "Oxford_MNK_Omega_Sign.vi"("error in (no error)"=w1051) -> ("error out"=w1050:errorcluster)  [unwired: 10 in]
        n464 = call <vilib>:"Add State(s) to Queue__JKI_lib_State_Machine.vi"("State(s) in (\"\")"=w1053) -> ("States Out"=w1054:string)  [unwired: 14 in]
      }
    }
  }
  n465 = disable-structure shown="Disabled" {
    frame Disabled {
      (unwired) FALSE
      n466 = call-poly <instrlib>:"Configuration (Read).vi"() -> ()  [unwired: 3 in, 9 out]
      n467 = disable-structure shown="Disabled" {
        frame Disabled {
          n468 = property on="Fast/Slow Fill" class="Bool (strict)" props=["Val(Sgnl)"]() -> ()  [unwired: 3 in, 2 out]
        }
        frame Enabled {
        }
      }
      n469 = local read "PS Heat"() -> ()  [unwired: 1 in]
      n470 = local read "Lambda"() -> ()  [unwired: 1 in]
    }
    frame Enabled {
    }
  }
